vi "Process_NEECA_Data.vi"(4 "Vesta in":refnum<queue>, 7 "Upper Temperature Sensor":T1, 8 "error in (no error)":errorcluster, 9 "VestaTemperature Fixed":T2={"Water Heater Temp (°F)"=125, "Differential  (°F)"=25.0} {"Water Heater Temp (°F)" min=32 max=203}, 10 "Differential_Top":dbl=10.0 format="%#_13g", 11 "Data Cluster":T3={"Vesta Data Output"={"Temp_W_Raw_U"=0, "Temp_W_Raw_L"=0, "Temperature Water (F)"=0.0, "Temperature Water Compensated (F)"=0.0, "Temperature Ambient (F)"=0.0, "Setpoint Location (F)"=0.0, "Heat Request"="", "Fault Ram"="", "PWM DCDC Value"=0, "Pilot Voltage (mV)"=0.0, "Setpoint Actual (F)"=0.0, "Differential Actual (F)"=0.0, "Setpoint User (F)"=0.0, "Differential User (F)"=0.0, "Termperature FIltered -TCO (F)"=0.0, "Temp_C_Raw_1 - Sensor Voltage"="", "Temp_C_Raw_2 - Sensor Voltage"="", "Chamber Sensor Temperature (F)"=0.0, "LDO Base Temperature (F)"=0.0, "LDO Timer (sec)"=0, "Disabled (0)"=FALSE, "Warming (1)"=FALSE, "Heating (2)"=FALSE, "Cooling Data Write (3)"=FALSE, "Cooling (4)"=FALSE, "Data Read (5)"=FALSE, "N/A"=FALSE, "Temperature Trip (7)"=FALSE, "Burner"=FALSE}, "VestaTemperature"={"Water Heater Temp (°F)"=135, "Differential  (°F)"=10.0}, "Timer Application Data"={"Duty Cycle"={"Burner ON Time (Seconds)"=60.0, "Burner OFF Time (Seconds)"=60.0, "Main Burner Flag"=FALSE, "Burner Power Mode"=0, "Off Time Complete Flag"=0, "Heating_Cycle_Released_Flag"=0, "Damper Status"=0, "Damper Burner Seen Flag"=0}}, "Data Array"=[], "MW Output"={"TC1-Channel 021"=0.0, "TC2-Channel 022"=0.0, "TC3-Channel 023"=0.0, "TC4-Channel 024"=0.0, "TC5-Channel 025"=0.0, "TC6-Channel 026"=0.0, "TC7-Channel 017"=0.0, "TC8-Channel 028"=0.0, "TC9-Channel 029"=0.0, "TC10-Channel 030"=0.0, "TC Tree Average"=0.0, "TC DWN- Channel 027"=0.0, "RTDin-Channel 031"=0.0, "RTDout-Channel 032"=0.0, "RTDamb-Channel 033"=0.0, "PSI1-Channel 011"=0.0, "PSI2-Channel 012"=0.0, "PSI3-Channel 013"=0.0, "PSI4-Channel 014"=0.0, "UE State-Channel 015"=0.0, "LE State-Channel 016"=0.0, "Module 4 Relay Status Output"={"INTELLIFAUCET TEMP(T)/FLOW(F) (CH 041)"=FALSE, "INTELLIFAUCET READY (CH 042)"=FALSE, "INTELLIFAUCET START (CH 043)"=FALSE, "INTELLIFAUCET STOP (CH 044)"=FALSE, "MAIN POWER RELAY (CH 047)"=FALSE, "NOT USED (CH 045)"=FALSE, "NOT USED (CH 046)"=FALSE, "PURGE VALVE RELAY (CH 048)"=FALSE, "OUTLET VALVE RELAY (CH 049)"=FALSE, "INLET VALVE RELAY (CH 050)"=FALSE, "Intellifaucet (% Open)"=0.0, "Proportioning Valve (%Open)"=0.0, "Intellifaucet Temp Setpoint (F)"=0.0}}} {"VestaTemperature"."Water Heater Temp (°F)" min=32 max=203}) -> (0 "error out":errorcluster, 2 "Open_Damper":i32, 3 "Data Cluster Output":T3={"Vesta Data Output"={"Temp_W_Raw_U"=0, "Temp_W_Raw_L"=0, "Temperature Water (F)"=0.0, "Temperature Water Compensated (F)"=0.0, "Temperature Ambient (F)"=0.0, "Setpoint Location (F)"=0.0, "Heat Request"="", "Fault Ram"="", "PWM DCDC Value"=0, "Pilot Voltage (mV)"=0.0, "Setpoint Actual (F)"=0.0, "Differential Actual (F)"=0.0, "Setpoint User (F)"=0.0, "Differential User (F)"=0.0, "Termperature FIltered -TCO (F)"=0.0, "Temp_C_Raw_1 - Sensor Voltage"="", "Temp_C_Raw_2 - Sensor Voltage"="", "Chamber Sensor Temperature (F)"=0.0, "LDO Base Temperature (F)"=0.0, "LDO Timer (sec)"=0, "Disabled (0)"=FALSE, "Warming (1)"=FALSE, "Heating (2)"=FALSE, "Cooling Data Write (3)"=FALSE, "Cooling (4)"=FALSE, "Data Read (5)"=FALSE, "N/A"=FALSE, "Temperature Trip (7)"=FALSE, "Burner"=FALSE}, "VestaTemperature"={"Water Heater Temp (°F)"=135, "Differential  (°F)"=10.0}, "Timer Application Data"={"Duty Cycle"={"Burner ON Time (Seconds)"=60.0, "Burner OFF Time (Seconds)"=60.0, "Main Burner Flag"=FALSE, "Burner Power Mode"=0, "Off Time Complete Flag"=0, "Heating_Cycle_Released_Flag"=0, "Damper Status"=0, "Damper Burner Seen Flag"=0}}, "Data Array"=[], "MW Output"={"TC1-Channel 021"=0.0, "TC2-Channel 022"=0.0, "TC3-Channel 023"=0.0, "TC4-Channel 024"=0.0, "TC5-Channel 025"=0.0, "TC6-Channel 026"=0.0, "TC7-Channel 017"=0.0, "TC8-Channel 028"=0.0, "TC9-Channel 029"=0.0, "TC10-Channel 030"=0.0, "TC Tree Average"=0.0, "TC DWN- Channel 027"=0.0, "RTDin-Channel 031"=0.0, "RTDout-Channel 032"=0.0, "RTDamb-Channel 033"=0.0, "PSI1-Channel 011"=0.0, "PSI2-Channel 012"=0.0, "PSI3-Channel 013"=0.0, "PSI4-Channel 014"=0.0, "UE State-Channel 015"=0.0, "LE State-Channel 016"=0.0, "Module 4 Relay Status Output"={"INTELLIFAUCET TEMP(T)/FLOW(F) (CH 041)"=FALSE, "INTELLIFAUCET READY (CH 042)"=FALSE, "INTELLIFAUCET START (CH 043)"=FALSE, "INTELLIFAUCET STOP (CH 044)"=FALSE, "MAIN POWER RELAY (CH 047)"=FALSE, "NOT USED (CH 045)"=FALSE, "NOT USED (CH 046)"=FALSE, "PURGE VALVE RELAY (CH 048)"=FALSE, "OUTLET VALVE RELAY (CH 049)"=FALSE, "INLET VALVE RELAY (CH 050)"=FALSE, "Intellifaucet (% Open)"=0.0, "Proportioning Valve (%Open)"=0.0, "Intellifaucet Temp Setpoint (F)"=0.0}}} {"VestaTemperature"."Water Heater Temp (°F)" min=32 max=203})   [LabVIEW 2023]
uses:
  Message Queue/Message Cluster.ctl
  controls/UI Data.ctl
  Drivers/Resideo Gas Valve/Type Definitions/Vesta Info.ctl
  Drivers/Resideo Gas Valve/Type Definitions/Temperature Control.ctl
  controls/Timer Application Cluster.ctl
  controls/Burner Duty Cycle.ctl
  Hybrid Water Heater/Type Definitions/HEWH MW100 Data Cluster.ctl
  Hybrid Water Heater/Custom Instrument Control/MW100/Type Definitions/HEWH Module 4 Relay Status.ctl
  controls/Upper Temperature Sensor.ctl
  <vilib>/Utility/error.llb/whitespace.ctl
  <vilib>/Utility/error.llb/Trim Whitespace One-Sided.vi
  Message Queue/Message Queue.lvlib
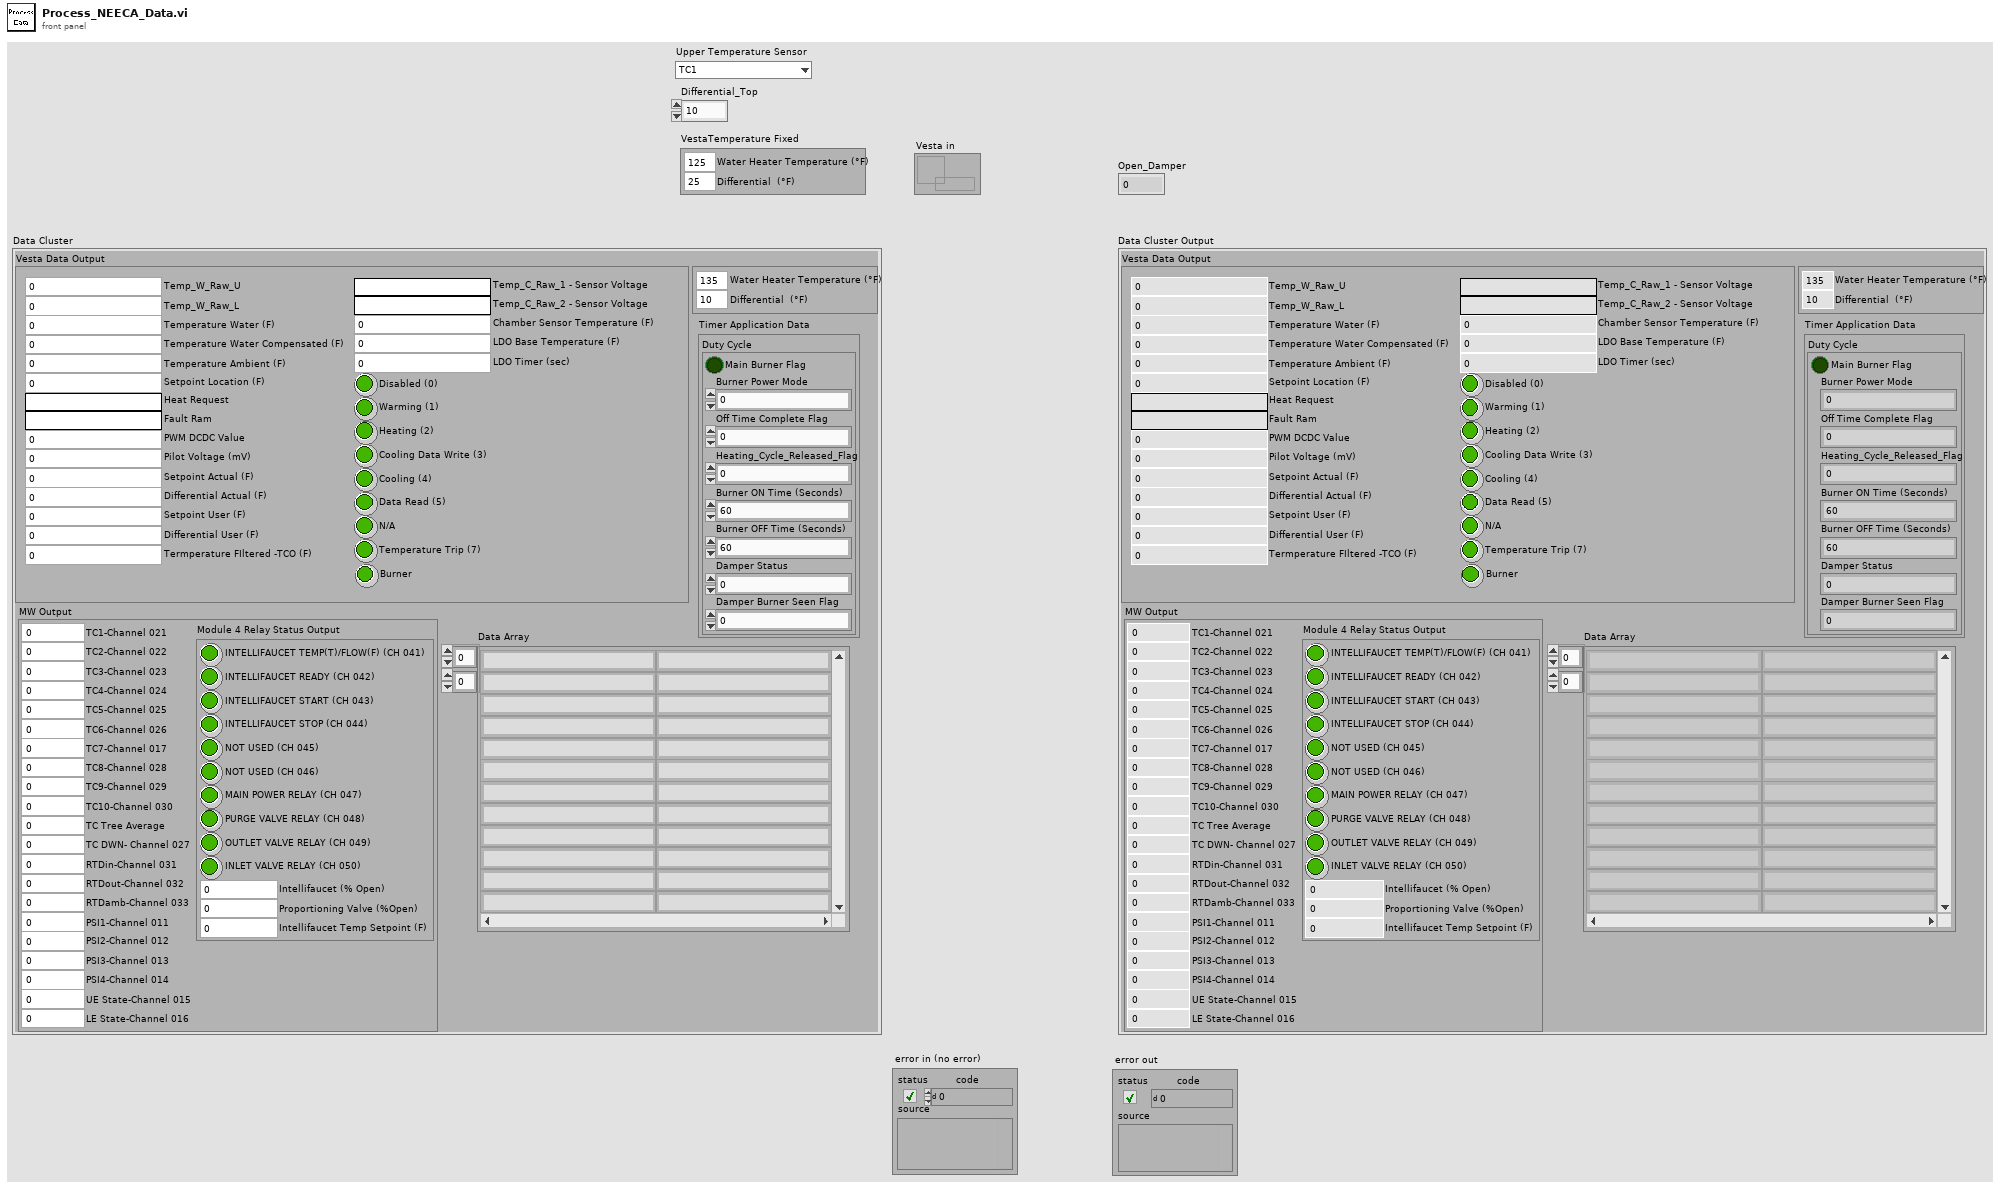
[diagram p1: front panel]
types:
  T1 = typedef "Upper Temperature Sensor.ctl" = enum16{"TC1", "TC2", "TC3", "TC4", "TC5", "TC6"}
  T2 = typedef "Temperature Control.ctl" = cluster{"Water Heater Temp (°F)":u16, "Differential  (°F)":dbl}
  T3 = typedef "UI Data.ctl" = cluster{"Vesta Data Output":T4, "VestaTemperature":T2, "Timer Application Data":T5, "Data Array":string[][], "MW Output":T7}
  T4 = typedef "Vesta Info.ctl" = cluster{"Temp_W_Raw_U":u16, "Temp_W_Raw_L":u16, "Temperature Water (F)":dbl, "Temperature Water Compensated (F)":dbl, "Temperature Ambient (F)":dbl, "Setpoint Location (F)":dbl, "Heat Request":string, "Fault Ram":string, "PWM DCDC Value":u16, "Pilot Voltage (mV)":dbl, "Setpoint Actual (F)":dbl, "Differential Actual (F)":dbl, "Setpoint User (F)":dbl, "Differential User (F)":dbl, "Termperature FIltered -TCO (F)":dbl, "Temp_C_Raw_1 - Sensor Voltage":string, "Temp_C_Raw_2 - Sensor Voltage":string, "Chamber Sensor Temperature (F)":dbl, "LDO Base Temperature (F)":dbl, "LDO Timer (sec)":i16, "Disabled (0)":bool, "Warming (1)":bool, "Heating (2)":bool, "Cooling Data Write (3)":bool, "Cooling (4)":bool, "Data Read (5)":bool, "N/A":bool, "Temperature Trip (7)":bool, "Burner":bool}
  T5 = typedef "Timer Application Cluster.ctl" = cluster{"Duty Cycle":T6}
  T6 = typedef "Burner Duty Cycle.ctl" = cluster{"Burner ON Time (Seconds)":dbl, "Burner OFF Time (Seconds)":dbl, "Main Burner Flag":bool, "Burner Power Mode":u8, "Off Time Complete Flag":u8, "Heating_Cycle_Released_Flag":u8, "Damper Status":u8, "Damper Burner Seen Flag":u8}
  T7 = typedef "HEWH MW100 Data Cluster.ctl" = cluster{"TC1-Channel 021":dbl, "TC2-Channel 022":dbl, "TC3-Channel 023":dbl, "TC4-Channel 024":dbl, "TC5-Channel 025":dbl, "TC6-Channel 026":dbl, "TC7-Channel 017":dbl, "TC8-Channel 028":dbl, "TC9-Channel 029":dbl, "TC10-Channel 030":dbl, "TC Tree Average":dbl, "TC DWN- Channel 027":dbl, "RTDin-Channel 031":dbl, "RTDout-Channel 032":dbl, "RTDamb-Channel 033":dbl, "PSI1-Channel 011":dbl, "PSI2-Channel 012":dbl, "PSI3-Channel 013":dbl, "PSI4-Channel 014":dbl, "UE State-Channel 015":dbl, "LE State-Channel 016":dbl, "Module 4 Relay Status Output":T8}
  T8 = typedef "HEWH Module 4 Relay Status.ctl" = cluster{"INTELLIFAUCET TEMP(T)/FLOW(F) (CH 041)":bool, "INTELLIFAUCET READY (CH 042)":bool, "INTELLIFAUCET START (CH 043)":bool, "INTELLIFAUCET STOP (CH 044)":bool, "MAIN POWER RELAY (CH 047)":bool, "NOT USED (CH 045)":bool, "NOT USED (CH 046)":bool, "PURGE VALVE RELAY (CH 048)":bool, "OUTLET VALVE RELAY (CH 049)":bool, "INLET VALVE RELAY (CH 050)":bool, "Intellifaucet (% Open)":dbl, "Proportioning Valve (%Open)":dbl, "Intellifaucet Temp Setpoint (F)":dbl}
  T9 = typedef "whitespace.ctl" = u16
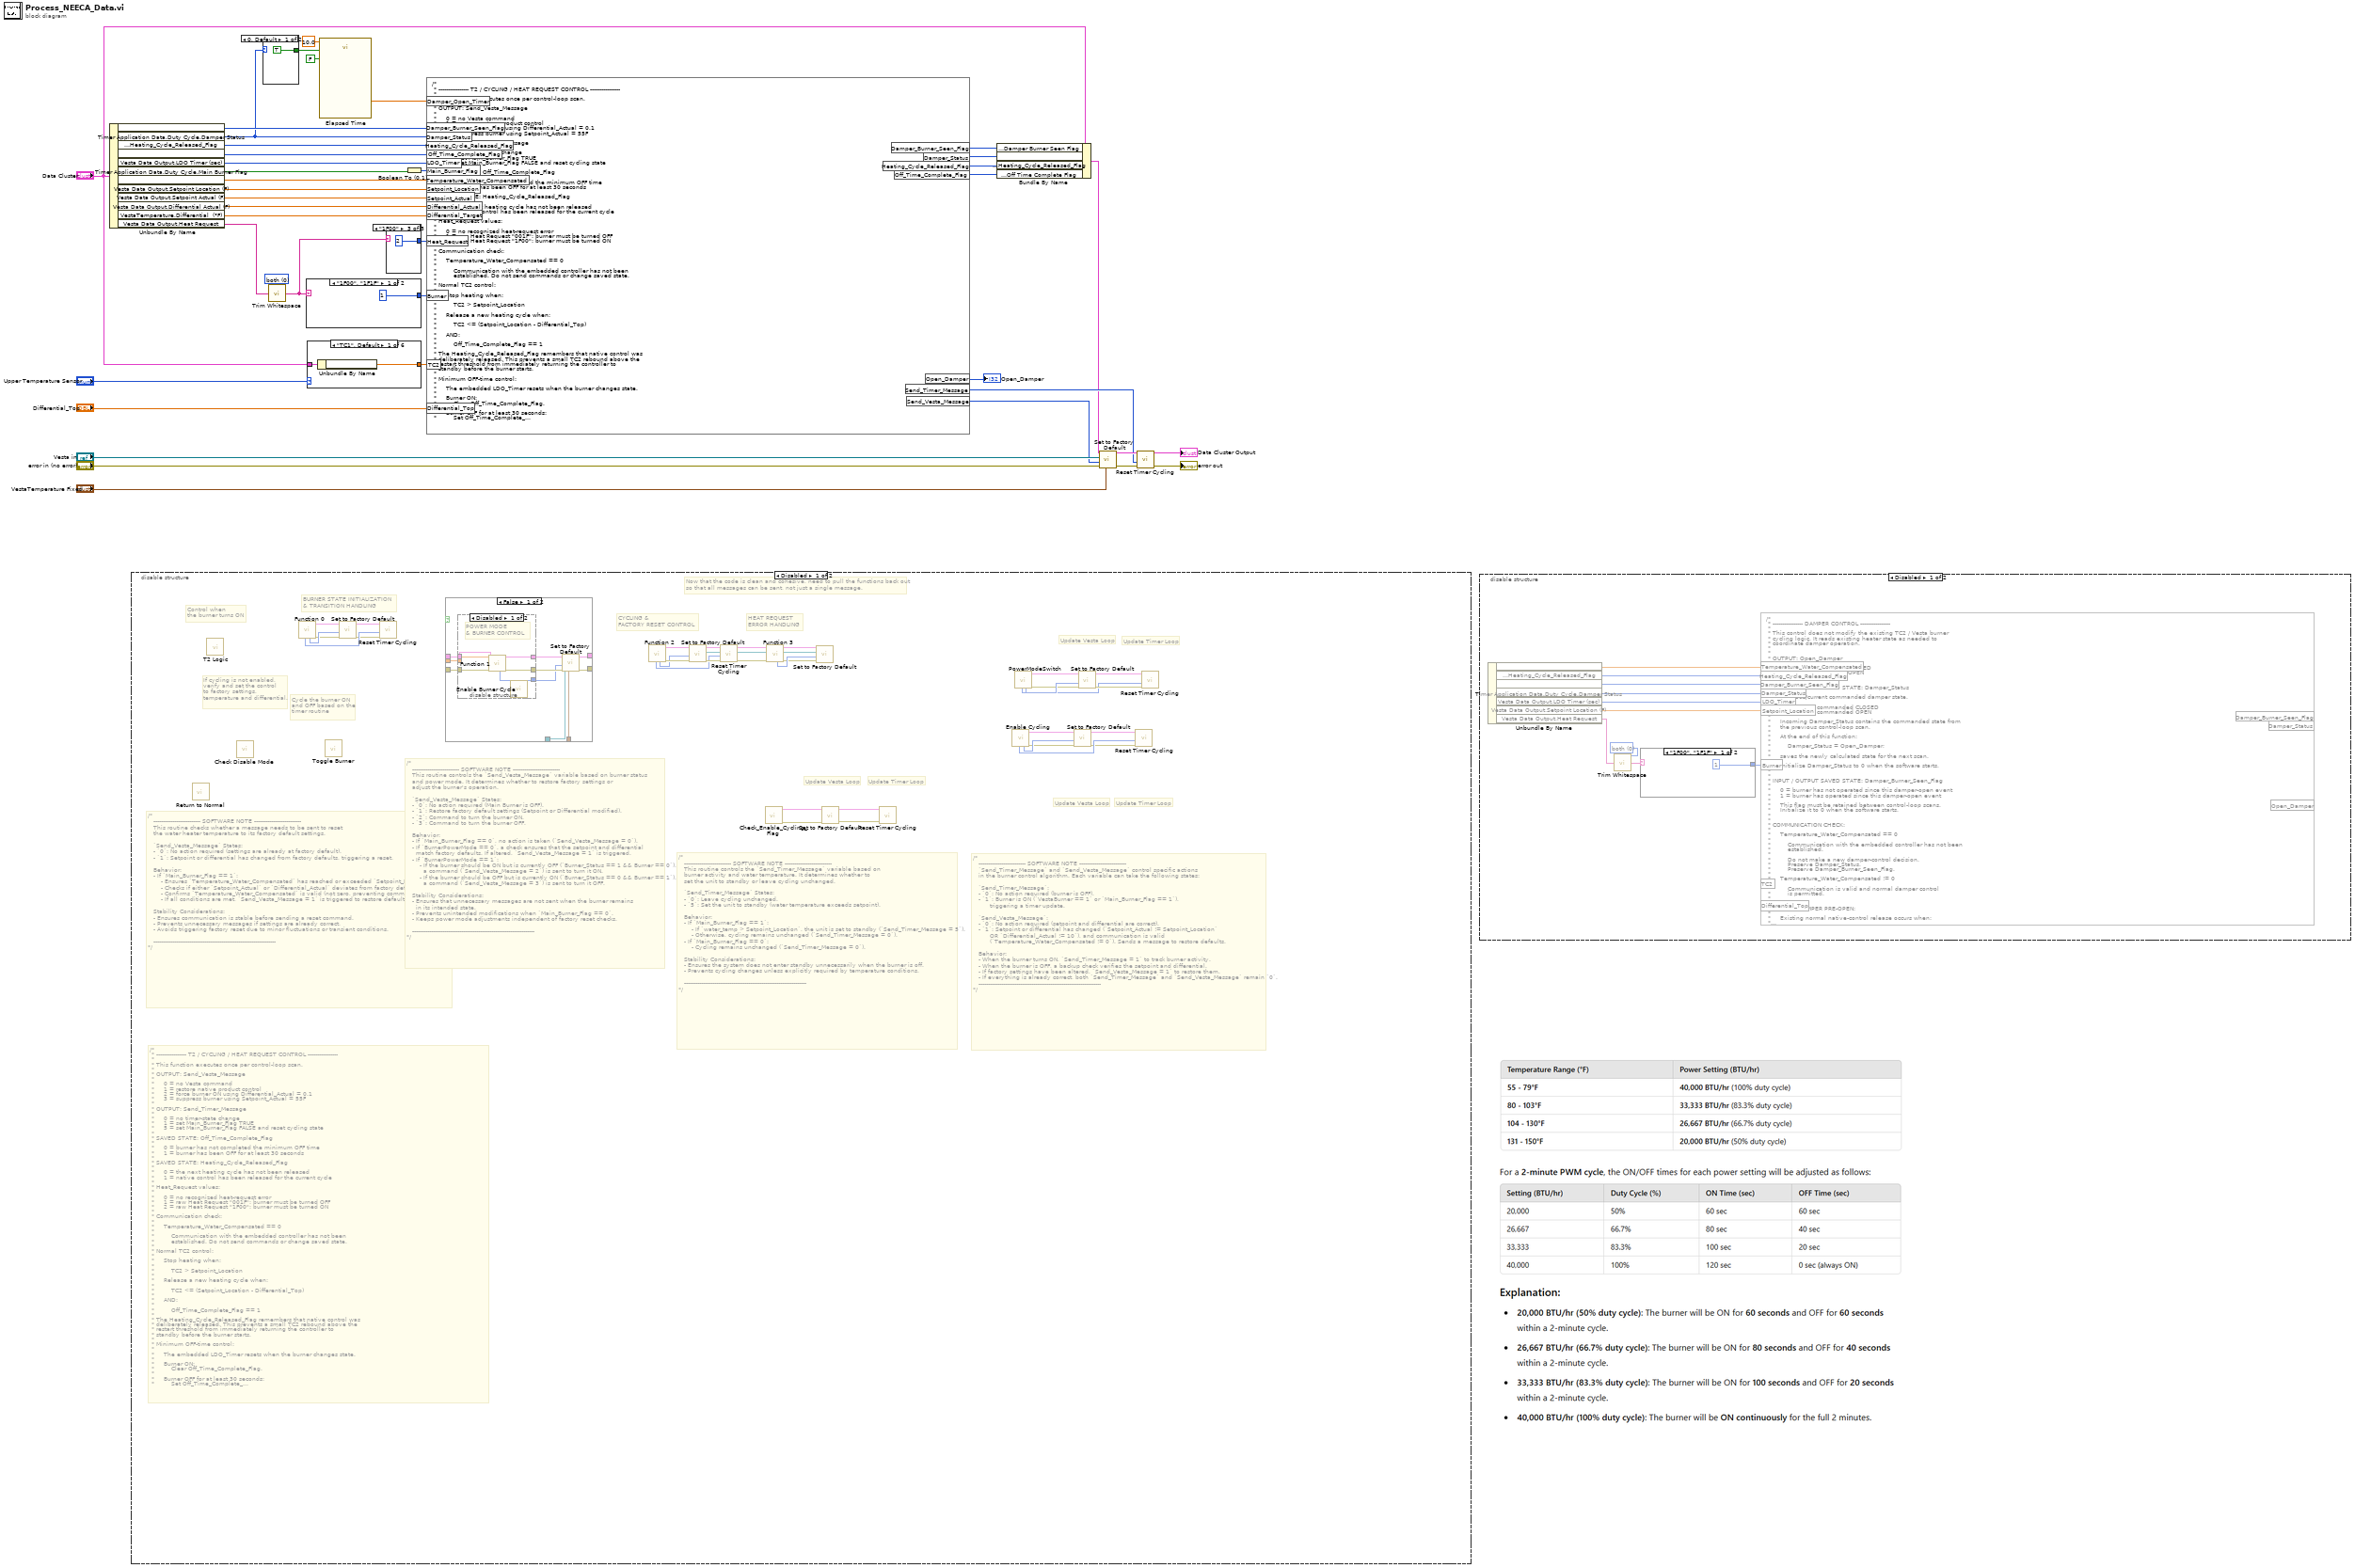
[diagram p0: block diagram]
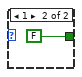
[diagram p2: hidden frame]
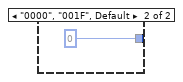
[diagram p3: hidden frame]
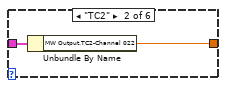
[diagram p5: hidden frame]
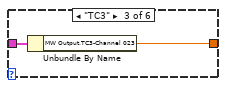
[diagram p6: hidden frame]
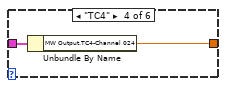
[diagram p7: hidden frame]
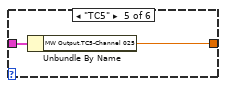
[diagram p8: hidden frame]
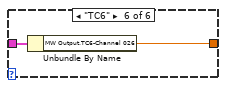
[diagram p9: hidden frame]
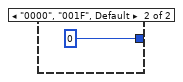
[diagram p10: hidden frame]
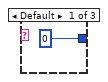
[diagram p11: hidden frame]
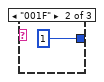
[diagram p12: hidden frame]
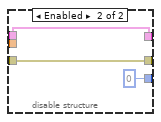
[diagram p13: hidden frame]
diagram:
  w27 = T9 0 items=["both", "start of string", "end of string"] ("location (both)")
  n1 = Unbundle By Name("Data Cluster") -> ("Timer Application Data.Duty Cycle.Damper Burner Seen Flag"=w9:u8, "Timer Application Data.Duty Cycle.Damper Status"=w3:u8, "Timer Application Data.Duty Cycle.Heating_Cycle_Released_Flag"=w14:u8, "Timer Application Data.Duty Cycle.Off Time Complete Flag"=w18:u8, "Vesta Data Output.LDO Timer (sec)"=w19:i16, "Timer Application Data.Duty Cycle.Main Burner Flag"=w24:bool, "Vesta Data Output.Temperature Water Compensated (F)"=w36:dbl, "Vesta Data Output.Setpoint Location (F)"=w31:dbl, "Vesta Data Output.Setpoint Actual (F)"=w30:dbl, "Vesta Data Output.Differential Actual (F)"=w29:dbl, "VestaTemperature.Differential  (°F)"=w28:dbl, "Vesta Data Output.Heat Request"=w26:string)
  n2 = disable-structure shown="Disabled" {
    frame Disabled {
      # "/*\n * ---------------- T2 / CYCLING / HEAT REQUEST CONTROL ----------------\n *\n * This function executes once per control-loop scan.\n *\n * OUTPUT: Send_Vesta_Message\n *\n *     0 = no Vesta command\n *     1 = restore native product control\n *     2 = force burner ON using Differential_Actual = 0.1\n *     3 = suppress burner using Setpoint_Actual = 55F\n *\n * OUTPUT: Send_Timer_Message\n *\n *     0 = no timer-state change\n *     1 = set Main_Burner_Flag TRUE\n *     5 = set Main_Burner_Flag FALSE and reset cycling state\n *\n * SAVED STATE: Off_Time_Complete_Flag\n *\n *     0 = burner has not completed the minimum OFF time\n *     1 = burner has been OFF for at least 30 seconds\n *\n * SAVED STATE: Heating_Cycle_Released_Flag\n *\n *     0 = the next heating cycle has not been released\n *     1 = native control has been released for the current cycle\n *\n * Heat_Request values:\n *\n *     0 = no recognized heat-request error\n *     1 = raw Heat Request \"001F\": burner must be turned OFF\n *     2 = raw Heat Request \"1F00\": burner must be turned ON\n *\n * Communication check:\n *\n *     Temperature_Water_Compensated == 0\n *\n *         Communication with the embedded controller has not been\n *         established. Do not send commands or change saved state.\n *\n * Normal TC2 control:\n *\n *     Stop heating when:\n *\n *         TC2 > Setpoint_Location\n *\n *     Release a new heating cycle when:\n *\n *         TC2 <= (Setpoint_Location - Differential_Top)\n *\n *     AND:\n *\n *         Off_Time_Complete_Flag == 1\n *\n * The Heating_Cycle_Released_Flag remembers that native control was\n * deliberately released. This prevents a small TC2 rebound above the\n * restart threshold from immediately returning the controller to\n * standby before the burner starts.\n *\n * Minimum OFF-time control:\n *\n *     The embedded LDO_Timer resets when the burner changes state.\n *\n *     Burner ON:\n *         Clear Off_Time_Complete_Flag.\n *\n *     Burner OFF for at least 30 seconds:\n *         Set Off_Time_Complete_Flag.\n *\n *     Once set, the flag stays set throughout the same OFF period.\n *     This prevents LDO_Timer rollover from restarting the lockout.\n *\n * Forced-ON error recovery:\n *\n *     Heat_Request == 2 applies Differential_Actual = 0.1.\n *\n *     After Heat_Request returns to zero, remove the 0.1 differential\n *     immediately. Do not wait for the TC2 restart threshold or the\n *     30-second OFF-time requirement.\n *\n * Control priority:\n *\n *     0. Embedded communication check\n *     1. Active Heat Request error handling\n *     2. Residual forced-ON error recovery\n *     3. Pilot position\n *     4. Normal TC2 cycle-release control\n */\n\n\n/* ---------------- Output defaults ---------------- */\n\nint32 Send_Vesta_Message = 0;\nint32 Send_Timer_Message = 0;\nint32 Open_Damper = 0;\n\n\n/* ---------------- Controller-state variables ---------------- */\n\nint32 native_controls_active = 0;\nint32 standby_is_active = 0;\nint32 forced_on_is_active = 0;\n\n\n/* ---------------- Communication and TC2 variables ---------------- */\n\nint32 lower_temperature_valid = 0;\nint32 upper_is_high = 0;\nint32 upper_restart_allowed = 0;\n\n\n/* ---------------- Previous saved-state values ---------------- */\n\nint32 Off_Time_Complete_Flag_Previous = 0;\nint32 Heating_Cycle_Released_Flag_Previous = 0;\n\n\n/* ---------------- Constants ---------------- */\n\nfloat Pilot_Position = 0.1;\nfloat Forced_On_Differential = 0.1;\n\nint32 LDO_Timeout_OFF = 30;\n\n\n/* ---------------- Decoded Heat Request values ---------------- */\n\nint32 Heat_Request_None = 0;\nint32 Heat_Request_Turn_Off = 1;  /* Raw value \"001F\" */\nint32 Heat_Request_Turn_On = 2;   /* Raw value \"1F00\" */\n\n\n/* ================================================================\n * SAVE INCOMING STATE VALUES\n * ================================================================ */\n\n/*\n * Both saved-state variables are Formula Node inputs and outputs.\n *\n * Preserve the incoming values by default. The control logic below\n * changes them only when a defined state transition occurs.\n */\n\nOff_Time_Complete_Flag_Previous =\n    Off_Time_Complete_Flag;\n\nHeating_Cycle_Released_Flag_Previous =\n    Heating_Cycle_Released_Flag;\n\nOff_Time_Complete_Flag =\n    Off_Time_Complete_Flag_Previous;\n\nHeating_Cycle_Released_Flag =\n    Heating_Cycle_Released_Flag_Previous;\n\n\n/* ================================================================\n * DETERMINE CURRENT EMBEDDED CONTROLLER STATE\n * ================================================================ */\n\n/*\n * Native control:\n *\n *     Setpoint_Actual = physical knob setting\n *     Differential_Actual = normal embedded differential\n */\n\nnative_controls_active =\n    ((Setpoint_Actual == Setpoint_Location) &&\n     (Differential_Actual == Differential_Target)) ? 1 : 0;\n\n\n/*\n * Standby:\n *\n *     Setpoint_Actual = 55F\n *     Differential_Actual = normal embedded differential\n */\n\nstandby_is_active =\n    ((Setpoint_Actual == 55.0) &&\n     (Differential_Actual == Differential_Target)) ? 1 : 0;\n\n\n/*\n * Forced ON:\n *\n *     Setpoint_Actual = physical knob setting\n *     Differential_Actual = 0.1\n */\n\nforced_on_is_active =\n    ((Setpoint_Actual == Setpoint_Location) &&\n     (Differential_Actual == Forced_On_Differential)) ? 1 : 0;\n\n\n/* ================================================================\n * DETERMINE COMMUNICATION STATUS\n * ================================================================ */\n\n/*\n * Temperature_Water_Compensated is used only as the communication\n * check in this function.\n *\n * A value of zero indicates that a valid reading has not been\n * received from the embedded controller.\n */\n\nlower_temperature_valid =\n    (Temperature_Water_Compensated == 0) ? 0 : 1;\n\n\n/* ================================================================\n * DETERMINE TC2 CONDITIONS\n * ================================================================ */\n\n/*\n * Stop heating when TC2 rises above the physical knob setpoint.\n *\n * At exact equality, upper_is_high remains zero.\n */\n\nupper_is_high =\n    (TC2 > Setpoint_Location) ? 1 : 0;\n\n\n/*\n * Permit release of a new heating cycle after TC2 cools to or below:\n *\n *     Setpoint_Location - Differential_Top\n *\n * Example:\n *\n *     Setpoint_Location = 125F\n *     Differential_Top = 5F\n *\n *     Stop threshold:    TC2 > 125F\n *     Restart threshold: TC2 <= 120F\n */\n\nupper_restart_allowed =\n    (TC2 <=\n        (Setpoint_Location - Differential_Top)) ? 1 : 0;\n\n\n/* ================================================================\n * PRIORITY 0: EMBEDDED COMMUNICATION CHECK\n * ================================================================ */\n\nif (lower_temperature_valid == 0)\n{\n    /*\n     * Communication has not been established.\n     *\n     * Do not send Vesta commands.\n     * Do not send timer commands.\n     * Do not change either saved-state flag.\n     */\n\n    Send_Vesta_Message = 0;\n    Send_Timer_Message = 0;\n\n    Off_Time_Complete_Flag =\n        Off_Time_Complete_Flag_Previous;\n\n    Heating_Cycle_Released_Flag =\n        Heating_Cycle_Released_Flag_Previous;\n}\n\n\n/* ================================================================\n * COMMUNICATION IS VALID\n * ================================================================ */\n\nelse\n{\n    /* ------------------------------------------------------------\n     * UPDATE MINIMUM OFF-TIME STATE\n     * ------------------------------------------------------------ */\n\n    /*\n     * Burner ON:\n     *\n     * The burner is no longer in an OFF period. Clear the completed\n     * OFF-time flag.\n     */\n\n    if (Burner == 1)\n    {\n        Off_Time_Complete_Flag = 0;\n    }\n\n\n    /*\n     * Burner OFF:\n     *\n     * Set the completed flag after LDO_Timer reaches 30 seconds.\n     *\n     * Once set, preserve the flag throughout the same OFF period.\n     * LDO_Timer may later roll over, but the saved flag stays set.\n     */\n\n    else if (Burner == 0)\n    {\n        if (Off_Time_Complete_Flag_Previous == 0)\n        {\n            if (LDO_Timer >= LDO_Timeout_OFF)\n            {\n                Off_Time_Complete_Flag = 1;\n            }\n        }\n    }\n\n\n    /*\n     * Unexpected burner value:\n     *\n     * Preserve the previous OFF-time state.\n     */\n\n    else\n    {\n        Off_Time_Complete_Flag =\n            Off_Time_Complete_Flag_Previous;\n    }\n\n\n    /* ============================================================\n     * PRIORITY 1A: ACTIVE TURN-OFF ERROR\n     * ============================================================ */\n\n    /*\n     * Heat_Request == 1 corresponds to raw value \"001F\".\n     *\n     * The error condition requires the burner to be turned OFF.\n     */\n\n    if (Heat_Request == Heat_Request_Turn_Off)\n    {\n        /*\n         * Immediately command 55F standby.\n         *\n         * Vesta message 3 also restores:\n         *\n         *     Differential_Actual = Differential_Target\n         */\n\n        if (standby_is_active == 0)\n        {\n            Send_Vesta_Message = 3;\n        }\n\n        /*\n         * Withdraw normal-cycle permission.\n         *\n         * After the error clears, the next normal cycle must satisfy\n         * the TC2 restart and minimum OFF-time requirements.\n         */\n\n        Heating_Cycle_Released_Flag = 0;\n\n        /*\n         * Do not clear Main_Burner_Flag until Burner == 0 confirms\n         * that the burner has physically shut down.\n         */\n    }\n\n\n    /* ============================================================\n     * PRIORITY 1B: ACTIVE FORCED-ON ERROR\n     * ============================================================ */\n\n    /*\n     * Heat_Request == 2 corresponds to raw value \"1F00\".\n     *\n     * The error condition requires the burner to be turned ON.\n     */\n\n    else if (Heat_Request == Heat_Request_Turn_On)\n    {\n        /*\n         * Immediately apply the 0.1 embedded lower differential.\n         *\n         * Active error handling is not delayed by TC2 restart\n         * permission or the 30-second minimum OFF time.\n         */\n\n        if (forced_on_is_active == 0)\n        {\n            Send_Vesta_Message = 2;\n        }\n\n        /*\n         * Preserve Heating_Cycle_Released_Flag while the active error\n         * is present.\n         *\n         * The residual forced-ON recovery below determines the proper\n         * normal state after Heat_Request returns to zero.\n         */\n    }\n\n\n    /* ============================================================\n     * PRIORITY 2: NO ACTIVE HEAT REQUEST ERROR\n     * ============================================================ */\n\n    else if (Heat_Request == Heat_Request_None)\n    {\n        /* --------------------------------------------------------\n         * RESIDUAL FORCED-ON ERROR RECOVERY\n         * -------------------------------------------------------- */\n\n        /*\n         * Heat_Request has cleared, but the controller still reports:\n         *\n         *     Setpoint_Actual = Setpoint_Location\n         *     Differential_Actual = 0.1\n         *\n         * Remove the 0.1 differential immediately.\n         *\n         * Do not wait for:\n         *\n         *     upper_restart_allowed\n         *     Off_Time_Complete_Flag\n         */\n\n        if (forced_on_is_active == 1)\n        {\n            /*\n             * TC2 is above the customer setpoint.\n             *\n             * Enter standby immediately and withdraw heating-cycle\n             * permission.\n             */\n\n            if (upper_is_high == 1)\n            {\n                Send_Vesta_Message = 3;\n                Heating_Cycle_Released_Flag = 0;\n            }\n\n\n            /*\n             * TC2 is not above the customer setpoint.\n             *\n             * Immediately restore:\n             *\n             *     Setpoint_Actual = Setpoint_Location\n             *     Differential_Actual = Differential_Target\n             *\n             * Consider the current cycle released. The embedded lower\n             * thermistor then decides whether the burner continues,\n             * shuts off, or starts later.\n             */\n\n            else\n            {\n                Send_Vesta_Message = 1;\n                Heating_Cycle_Released_Flag = 1;\n            }\n\n\n            /*\n             * Synchronize Main_Burner_Flag with the physical burner.\n             */\n\n            if (Burner == 1)\n            {\n                if (Main_Burner_Flag == 0)\n                {\n                    Send_Timer_Message = 1;\n                }\n            }\n\n            else if (Burner == 0)\n            {\n                if (Main_Burner_Flag == 1)\n                {\n                    Send_Timer_Message = 5;\n                }\n            }\n        }\n\n\n        /* --------------------------------------------------------\n         * USER-SELECTED PILOT POSITION\n         * -------------------------------------------------------- */\n\n        else if (Setpoint_Location == Pilot_Position)\n        {\n            /*\n             * Pilot was selected using the physical product control.\n             *\n             * Do not send Vesta or timer commands.\n             * Withdraw normal heating-cycle permission so that the\n             * control initializes again after leaving Pilot.\n             */\n\n            Send_Vesta_Message = 0;\n            Send_Timer_Message = 0;\n\n            Heating_Cycle_Released_Flag = 0;\n        }\n\n\n        /* --------------------------------------------------------\n         * BURNER ON\n         * -------------------------------------------------------- */\n\n        else if (Burner == 1)\n        {\n            /*\n             * TC2 is above the physical knob setpoint.\n             *\n             * Stop heating immediately regardless of release state.\n             */\n\n            if (upper_is_high == 1)\n            {\n                if (standby_is_active == 0)\n                {\n                    Send_Vesta_Message = 3;\n                }\n\n                /*\n                 * Withdraw permission for the next heating cycle.\n                 */\n\n                Heating_Cycle_Released_Flag = 0;\n\n                /*\n                 * Do not clear Main_Burner_Flag yet.\n                 *\n                 * Wait for Burner == 0 to confirm physical shutdown.\n                 */\n            }\n\n\n            /*\n             * A normal cycle was previously released.\n             *\n             * Continue heating while TC2 remains at or below the\n             * upper stopping threshold.\n             */\n\n            else if (Heating_Cycle_Released_Flag_Previous == 1)\n            {\n                Heating_Cycle_Released_Flag = 1;\n\n                if (Main_Burner_Flag == 0)\n                {\n                    Send_Timer_Message = 1;\n                }\n            }\n\n\n            /*\n             * Burner is already ON, but no released cycle has yet\n             * been recorded.\n             *\n             * This can happen during:\n             *\n             *     Cold-tank startup\n             *     Software restart\n             *     State recovery\n             *\n             * Adopt the active cycle only when TC2 is already at or\n             * below the normal restart threshold.\n             */\n\n            else\n            {\n                if (upper_restart_allowed == 1)\n                {\n                    /*\n                     * Adopt the valid cold-start heating cycle.\n                     */\n\n                    Heating_Cycle_Released_Flag = 1;\n\n                    /*\n                     * If the controller is not already in native mode,\n                     * restore native settings.\n                     */\n\n                    if (native_controls_active == 0)\n                    {\n                        Send_Vesta_Message = 1;\n                    }\n\n                    if (Main_Burner_Flag == 0)\n                    {\n                        Send_Timer_Message = 1;\n                    }\n                }\n\n\n                /*\n                 * The burner is ON, but TC2 is still above the restart\n                 * threshold.\n                 *\n                 * Do not adopt this cycle. Command standby and keep the\n                 * cycle locked out.\n                 */\n\n                else\n                {\n                    if (standby_is_active == 0)\n                    {\n                        Send_Vesta_Message = 3;\n                    }\n\n                    Heating_Cycle_Released_Flag = 0;\n                }\n            }\n        }\n\n\n        /* --------------------------------------------------------\n         * BURNER OFF\n         * -------------------------------------------------------- */\n\n        else if (Burner == 0)\n        {\n            /*\n             * Clear Main_Burner_Flag only after physical burner\n             * shutdown is confirmed.\n             */\n\n            if (Main_Burner_Flag == 1)\n            {\n                Send_Timer_Message = 5;\n            }\n\n\n            /*\n             * A cycle was previously released.\n             */\n\n            if (Heating_Cycle_Released_Flag_Previous == 1)\n            {\n                /*\n                 * TC2 has exceeded the customer setpoint while the\n                 * burner is OFF.\n                 *\n                 * Enter standby and close the released cycle.\n                 */\n\n                if (upper_is_high == 1)\n                {\n                    if (standby_is_active == 0)\n                    {\n                        Send_Vesta_Message = 3;\n                    }\n\n                    Heating_Cycle_Released_Flag = 0;\n                }\n\n\n                /*\n                 * Main_Burner_Flag is still one while Burner is zero.\n                 *\n                 * The embedded controller has just ended an active\n                 * burner cycle. Enter standby and require the next\n                 * cycle to satisfy TC2 and minimum OFF-time criteria.\n                 */\n\n                else if (Main_Burner_Flag == 1)\n                {\n                    if (standby_is_active == 0)\n                    {\n                        Send_Vesta_Message = 3;\n                    }\n\n                    Heating_Cycle_Released_Flag = 0;\n                }\n\n\n                /*\n                 * The cycle has been released, but the burner has not\n                 * started yet.\n                 *\n                 * Keep native control released while waiting for the\n                 * embedded lower thermistor to call for heat.\n                 *\n                 * Do not cancel the release merely because TC2 rises\n                 * slightly above the restart threshold.\n                 */\n\n                else\n                {\n                    Heating_Cycle_Released_Flag = 1;\n\n                    /*\n                     * If message 1 has not yet been acknowledged and\n                     * standby still reports active, repeat the same\n                     * release command. Do not issue an opposing\n                     * standby command.\n                     */\n\n                    if (standby_is_active == 1)\n                    {\n                        Send_Vesta_Message = 1;\n                    }\n\n                    else\n                    {\n                        Send_Vesta_Message = 0;\n                    }\n                }\n            }\n\n\n            /*\n             * No heating cycle is currently released.\n             */\n\n            else\n            {\n                /*\n                 * TC2 is above the physical knob setpoint.\n                 *\n                 * Ensure the controller is in standby.\n                 */\n\n                if (upper_is_high == 1)\n                {\n                    if (standby_is_active == 0)\n                    {\n                        Send_Vesta_Message = 3;\n                    }\n\n                    Heating_Cycle_Released_Flag = 0;\n                }\n\n\n                /*\n                 * The controller already reports standby.\n                 *\n                 * Release native control only after:\n                 *\n                 *     1. TC2 reaches the restart threshold.\n                 *     2. Burner has been OFF for at least 30 seconds.\n                 */\n\n                else if (standby_is_active == 1)\n                {\n                    if ((upper_restart_allowed == 1) &&\n                        (Off_Time_Complete_Flag == 1))\n                    {\n                        Send_Vesta_Message = 1;\n                        Heating_Cycle_Released_Flag = 1;\n                    }\n\n                    else\n                    {\n                        Send_Vesta_Message = 0;\n                        Heating_Cycle_Released_Flag = 0;\n                    }\n                }\n\n\n                /*\n                 * The controller reports native mode, but the cycle\n                 * has not yet been released.\n                 *\n                 * This is the startup and state-initialization case.\n                 */\n\n                else if (native_controls_active == 1)\n                {\n                    /*\n                     * Cold start or sufficiently cooled tank:\n                     *\n                     * Native control may remain active only after the\n                     * TC2 and minimum OFF-time criteria are satisfied.\n                     */\n\n                    if ((upper_restart_allowed == 1) &&\n                        (Off_Time_Complete_Flag == 1))\n                    {\n                        Send_Vesta_Message = 0;\n                        Heating_Cycle_Released_Flag = 1;\n                    }\n\n\n                    /*\n                     * Hot startup or minimum OFF time not complete:\n                     *\n                     * Place the controller into standby and lock out\n                     * the next heating cycle.\n                     */\n\n                    else\n                    {\n                        Send_Vesta_Message = 3;\n                        Heating_Cycle_Released_Flag = 0;\n                    }\n                }\n\n\n                /*\n                 * The applied state does not match native or standby.\n                 *\n                 * This may occur while a previous Vesta command is\n                 * still being processed. Do not issue an opposing\n                 * command.\n                 */\n\n                else\n                {\n                    Send_Vesta_Message = 0;\n                    Heating_Cycle_Released_Flag = 0;\n                }\n            }\n        }\n\n\n        /* --------------------------------------------------------\n         * UNEXPECTED BURNER VALUE\n         * -------------------------------------------------------- */\n\n        else\n        {\n            Send_Vesta_Message = 0;\n            Send_Timer_Message = 0;\n\n            Heating_Cycle_Released_Flag =\n                Heating_Cycle_Released_Flag_Previous;\n        }\n    }\n\n\n    /* ============================================================\n     * UNEXPECTED HEAT REQUEST VALUE\n     * ============================================================ */\n\n    else\n    {\n        Send_Vesta_Message = 0;\n        Send_Timer_Message = 0;\n\n        Heating_Cycle_Released_Flag =\n            Heating_Cycle_Released_Flag_Previous;\n    }\n}"
      # "Control when\nthe burner turns ON"
      # "CYCLING &\nFACTORY RESET CONTROL"
      # "HEAT REQUEST\nERROR HANDLING"
      # "BURNER STATE INITIALIZATION\n& TRANSITION HANDLING"
      # "Update Timer Loop"
      # "Update Vesta Loop"
      # "Now that the code is clean and cohesive, need to pull the functions back out\nso that all messages can be sent, not just a single message."
      # "/*  \n   ------------------------- SOFTWARE NOTE -------------------------  \n   `Send_Timer_Message` and `Send_Vesta_Message` control specific actions  \n   in the burner control algorithm. Each variable can take the following states:  \n\n   `Send_Timer_Message`:  \n   - `0`: No action required (burner is OFF).  \n   - `1`: Burner is ON (`VestaBurner == 1` or `Main_Burner_Flag == 1`),  \n         triggering a timer update.  \n\n   `Send_Vesta_Message`:  \n   - `0`: No action required (setpoint and differential are correct).  \n   - `1`: Setpoint or differential has changed (`Setpoint_Actual != Setpoint_Location`  \n         OR `Differential_Actual != 10`), and communication is valid  \n         (`Temperature_Water_Compensated != 0`). Sends a message to restore defaults.  \n\n   Behavior:  \n   - When the burner turns ON, `Send_Timer_Message = 1` to track burner activity.  \n   - When the burner is OFF, a backup check verifies the setpoint and differential.  \n   - If factory settings have been altered, `Send_Vesta_Message = 1` to restore them.  \n   - If everything is already correct, both `Send_Timer_Message` and `Send_Vesta_Message` remain `0`.  \n   -----------------------------------------------------------------  \n*/"
      # "Update Timer Loop"
      # "Update Vesta Loop"
      # "Update Timer Loop"
      # "Update Vesta Loop"
      # "/*  \n   ------------------------- SOFTWARE NOTE -------------------------  \n   This routine controls the `Send_Timer_Message` variable based on  \n   burner activity and water temperature. It determines whether to  \n   set the unit to standby or leave cycling unchanged.\n\n   `Send_Timer_Message` States:  \n   - `0`: Leave cycling unchanged.  \n   - `5`: Set the unit to standby (water temperature exceeds setpoint).  \n\n   Behavior:  \n   - If `Main_Burner_Flag == 1`:  \n       - If `water_temp > Setpoint_Location`, the unit is set to standby (`Send_Timer_Message = 5`).  \n       - Otherwise, cycling remains unchanged (`Send_Timer_Message = 0`).  \n   - If `Main_Burner_Flag == 0`:  \n       - Cycling remains unchanged (`Send_Timer_Message = 0`).  \n\n   Stability Considerations:  \n   - Ensures the system does not enter standby unnecessarily when the burner is off.  \n   - Prevents cycling changes unless explicitly required by temperature conditions.  \n\n   -----------------------------------------------------------------\n*/"
      # "/*  \n   ------------------------- SOFTWARE NOTE -------------------------  \n   This routine checks whether a message needs to be sent to reset  \n   the water heater temperature to its factory default settings.  \n\n   `Send_Vesta_Message` States:  \n   - `0`: No action required (settings are already at factory default).  \n   - `1`: Setpoint or differential has changed from factory defaults, triggering a reset.  \n\n   Behavior:  \n   - If `Main_Burner_Flag == 1`:  \n       - Ensures `Temperature_Water_Compensated` has reached or exceeded `Setpoint_Location`.  \n       - Checks if either `Setpoint_Actual` or `Differential_Actual` deviates from factory default.  \n       - Confirms `Temperature_Water_Compensated` is valid (not zero, preventing communication errors).  \n       - If all conditions are met, `Send_Vesta_Message = 1` is triggered to restore default settings.  \n\n   Stability Considerations:  \n   - Ensures communication is stable before sending a reset command.  \n   - Prevents unnecessary messages if settings are already correct.  \n   - Avoids triggering factory reset due to minor fluctuations or transient conditions.  \n\n   -----------------------------------------------------------------\n*/"
      # "/*  \n   ------------------------- SOFTWARE NOTE -------------------------  \n   This routine controls the `Send_Vesta_Message` variable based on burner status  \n   and power mode. It determines whether to restore factory settings or  \n   adjust the burner's operation.\n\n   `Send_Vesta_Message` States:  \n   - `0`: No action required (Main Burner is OFF).  \n   - `1`: Restore factory default settings (Setpoint or Differential modified).  \n   - `2`: Command to turn the burner ON.  \n   - `3`: Command to turn the burner OFF.  \n\n   Behavior:  \n   - If `Main_Burner_Flag == 0`, no action is taken (`Send_Vesta_Message = 0`).  \n   - If `BurnerPowerMode == 0`, a check ensures that the setpoint and differential  \n     match factory defaults. If altered, `Send_Vesta_Message = 1` is triggered.  \n   - If `BurnerPowerMode == 1`:  \n       - If the burner should be ON but is currently OFF (`Burner_Status == 1 && Burner == 0`),  \n         a command (`Send_Vesta_Message = 2`) is sent to turn it ON.  \n       - If the burner should be OFF but is currently ON (`Burner_Status == 0 && Burner == 1`),  \n         a command (`Send_Vesta_Message = 3`) is sent to turn it OFF.  \n\n   Stability Considerations:  \n   - Ensures that unnecessary messages are not sent when the burner remains  \n     in its intended state.  \n   - Prevents unintended modifications when `Main_Burner_Flag == 0`.  \n   - Keeps power mode adjustments independent of factory reset checks.  \n\n   -----------------------------------------------------------------\n*/"
      # "Cycle the burner ON\nand OFF based on the\ntimer routine"
      # "If cycling is not enabled,\nverify and set the control\nto factory settings,\ntemperature and differential."
      n3 = call "Return to Normal.vi"() -> ()  [unwired: 9 in, 3 out]
      n4 = call "T2 Logic.vi"() -> ()  [unwired: 8 in, 4 out]
      n5 = call "Check Disable Mode.vi"() -> ()  [unwired: 10 in, 2 out]
      n6 = call "Function 0.vi"() -> ("error out"=w55:errorcluster, "Data Cluster Out"=w56:T3, "Send_Vesta_Message"=w57:u8, "Send_Timer_Message"=w58:u8)  [unwired: 8 in]
      n7 = call "Toggle Burner.vi"() -> ()  [unwired: 10 in, 2 out]
      n8 = call "Set to Factory Default.vi"("error in (no error)"=w55, "Send_Vesta_Message"=w57, "Data Cluster In"=w56) -> ("error out"=w53:errorcluster, "Data Cluster Out"=w54:T3)  [unwired: 7 in]
      n9 = call "Reset Timer Cycling.vi"("error in (no error)"=w53, "Send_Timer_Message"=w58, "Data Cluster In"=w54) -> ()  [unwired: 7 in, 2 out]
      n10 = case shown="False" {
        selector: _ -> [_ _]
        tunnel: [w79 w94] -> _
        tunnel: [w80 w95] -> _
        tunnel: _ -> [w78 w95]
        tunnel: _ -> [w77 w94]
        tunnel: _ -> [w81 _]
        tunnel: _ -> [w76 _]
        tunnel: _ -> [w75 _]
        frame False {
          n11 = disable-structure shown="Disabled" {
            disable-tunnel: [w90 w92] -> w84
            disable-tunnel: [w89 w93] -> w83
            disable-tunnel: [w88 u8 0 ("Send_Vesta_Message")] -> w82
            disable-tunnel: w78 -> [w87 w93]
            disable-tunnel: w77 -> [w86 w92]
            disable-tunnel: w76 -> [w85 _]
            frame Disabled {
              # "POWER MODE\n& BURNER CONTROL"
              n12 = call "Function 1.vi"("error in (no error)"=w86, "Differential_Top"=w85, "Data Cluster"=w87) -> ("error out"=w90:errorcluster, "Data Cluster Out"=w89:T3, "Send_Vesta_Message"=w88:u8)  [unwired: 6 in]
            }
            frame Enabled {
            }
          }
          n13 = call "Set to Factory Default.vi"("VestaTemperature Fixed"=w75, "error in (no error)"=w84, "Send_Vesta_Message"=w82, "Vesta in"=w81, "Data Cluster In"=w83) -> ("error out"=w79:errorcluster, "Data Cluster Out"=w80:T3)  [unwired: 5 in]
        }
        frame True {
        }
      }
      n14 = call "Enable Burner Cycle.vi"() -> ()  [unwired: 9 in, 3 out]
      n15 = call "Function 2.vi"() -> ("error out"=w47:errorcluster, "Data Cluster Out"=w46:T3, "Send_Vesta_Message"=w44:u8, "Send_Timer_Message"=w45:u8)  [unwired: 8 in]
      n16 = call "Check_Enable_Cycling_Flag.vi"() -> ("error out"=w71:errorcluster, "Data Cluster out"=w72:T3)  [unwired: 8 in, 2 out]
      n17 = call "Set to Factory Default.vi"("error in (no error)"=w71, "Data Cluster In"=w72) -> ("error out"=w73:errorcluster, "Data Cluster Out"=w74:T3)  [unwired: 8 in]
      n18 = call "Reset Timer Cycling.vi"("error in (no error)"=w73, "Data Cluster In"=w74) -> ()  [unwired: 8 in, 2 out]
      n19 = call "Enable Cycling.vi"() -> ("error out"=w68:errorcluster, "Data Cluster out"=w67:T3, "Send_Vesta_Message"=w69:u8, "Send_Timer_Message"=w70:u8)  [unwired: 8 in]
      n20 = call "PowerModeSwitch.vi"() -> ("error out"=w60:errorcluster, "Data Cluster out"=w61:T3, "Send_Vesta_Message"=w64:u8, "Send_Timer_Message"=w59:u8)  [unwired: 8 in]
      n21 = call "Set to Factory Default.vi"("error in (no error)"=w68, "Send_Vesta_Message"=w69, "Data Cluster In"=w67) -> ("error out"=w66:errorcluster, "Data Cluster Out"=w65:T3)  [unwired: 7 in]
      n22 = call "Set to Factory Default.vi"("error in (no error)"=w60, "Send_Vesta_Message"=w64, "Data Cluster In"=w61) -> ("error out"=w63:errorcluster, "Data Cluster Out"=w62:T3)  [unwired: 7 in]
      n23 = call "Reset Timer Cycling.vi"("error in (no error)"=w66, "Send_Timer_Message"=w70, "Data Cluster In"=w65) -> ()  [unwired: 7 in, 2 out]
      n24 = call "Reset Timer Cycling.vi"("error in (no error)"=w63, "Send_Timer_Message"=w59, "Data Cluster In"=w62) -> ()  [unwired: 7 in, 2 out]
      n25 = call "Set to Factory Default.vi"("error in (no error)"=w47, "Send_Vesta_Message"=w44, "Vesta in"=w52, "Data Cluster In"=w46) -> ("error out"=w49:errorcluster, "Data Cluster Out"=w48:T3)  [unwired: 6 in]
      n26 = call "Reset Timer Cycling.vi"("error in (no error)"=w49, "Send_Timer_Message"=w45, "Data Cluster In"=w48) -> ("error out"=w50:errorcluster, "Data Cluster Output"=w51:T3)  [unwired: 7 in]
      n27 = call "Function 3.vi"("error in (no error)"=w50, "Data Cluster in"=w51) -> ("error out"=w41:errorcluster, "Data Cluster 3"=w42:T3, "Send_Vesta_Message"=w43:u8)  [unwired: 7 in]
      n28 = call "Set to Factory Default.vi"("error in (no error)"=w41, "Send_Vesta_Message"=w43, "Data Cluster In"=w42) -> ("Vesta in"=w52:refnum<queue>)  [unwired: 6 in, 2 out]
    }
    frame Enabled {
    }
  }
  n29 = case shown="0, Default" w3 {
    tunnel: [TRUE FALSE] -> w4
    frame 0, Default {
    }
    frame 1 {
    }
  }
  n30 = call <vilib>:"Trim Whitespace.vi"("string"=w26, "location (both)"=w27) -> ("trimmed string"=w22:string)
  n31 = case shown="\"1F00\", \"1F1F\"" w22 {
    tunnel: [1 0] -> w21
    frame "1F00", "1F1F" {
    }
    frame "0000", "001F", Default {
    }
  }
  n32 = case shown="\"TC1\", Default" "Upper Temperature Sensor" {
    tunnel: "Data Cluster" -> [w101 w103 w105 w107 w109 w111]
    tunnel: [w100 w102 w104 w106 w108 w110] -> w20
    frame "TC1", Default {
      n33 = Unbundle By Name(w101) -> ("MW Output.TC1-Channel 021"=w100:dbl)
    }
    frame "TC2" {
      n34 = Unbundle By Name(w103) -> ("MW Output.TC2-Channel 022"=w102:dbl)
    }
    frame "TC3" {
      n35 = Unbundle By Name(w105) -> ("MW Output.TC3-Channel 023"=w104:dbl)
    }
    frame "TC4" {
      n36 = Unbundle By Name(w107) -> ("MW Output.TC4-Channel 024"=w106:dbl)
    }
    frame "TC5" {
      n37 = Unbundle By Name(w109) -> ("MW Output.TC5-Channel 025"=w108:dbl)
    }
    frame "TC6" {
      n38 = Unbundle By Name(w111) -> ("MW Output.TC6-Channel 026"=w110:dbl)
    }
  }
  n39 = call "Elapsed Time"("Time Target (s)"=10.0, "Reset"=w4, "Auto Reset"=FALSE) -> ("Elapsed Time (s)"=w2:dbl)  [unwired: 9 in, 7 out]
  n40 = case shown="\"1F00\"" w22 {
    tunnel: [0 1 2] -> w25
    frame Default {
    }
    frame "001F" {
    }
    frame "1F00" {
    }
  }
  n41 = Boolean To (0,1)(Boolean=w24) -> (0, 1=w23:i16)
  n42 = formula code="/*\n * ---------------- T2 / CYCLING / HEAT REQUEST CONTROL ----------------\n *\n * This function executes once per control-loop scan.\n *\n * OUTPUT: Send_Vesta_Message\n *\n *     0 = no Vesta command\n *     1 = restore native product control\n *     2 = force burner ON using Differential_Actual = 0.1\n *     3 = suppress burner using Setpoint_Actual = 55F\n *\n * OUTPUT: Send_Timer_Message\n *\n *     0 = no timer-state change\n *     1 = set Main_Burner_Flag TRUE\n *     5 = set Main_Burner_Flag FALSE and reset cycling state\n *\n * SAVED STATE: Off_Time_Complete_Flag\n *\n *     0 = burner has not completed the minimum OFF time\n *     1 = burner has been OFF for at least 30 seconds\n *\n * SAVED STATE: Heating_Cycle_Released_Flag\n *\n *     0 = the next heating cycle has not been released\n *     1 = native control has been released for the current cycle\n *\n * Heat_Request values:\n *\n *     0 = no recognized heat-request error\n *     1 = raw Heat Request \"001F\": burner must be turned OFF\n *     2 = raw Heat Request \"1F00\": burner must be turned ON\n *\n * Communication check:\n *\n *     Temperature_Water_Compensated == 0\n *\n *         Communication with the embedded controller has not been\n *         established. Do not send commands or change saved state.\n *\n * Normal TC2 control:\n *\n *     Stop heating when:\n *\n *         TC2 > Setpoint_Location\n *\n *     Release a new heating cycle when:\n *\n *         TC2 <= (Setpoint_Location - Differential_Top)\n *\n *     AND:\n *\n *         Off_Time_Complete_Flag == 1\n *\n * The Heating_Cycle_Released_Flag remembers that native control was\n * deliberately released. This prevents a small TC2 rebound above the\n * restart threshold from immediately returning the controller to\n * standby before the burner starts.\n *\n * Minimum OFF-time control:\n *\n *     The embedded LDO_Timer resets when the burner changes state.\n *\n *     Burner ON:\n *         Clear Off_Time_Complete_Flag.\n *\n *     Burner OFF for at least 30 seconds:\n *         Set Off_Time_Complete_Flag.\n *\n *     Once set, the flag stays set throughout the same OFF period.\n *     This prevents LDO_Timer rollover from restarting the lockout.\n *\n * Forced-ON error recovery:\n *\n *     Heat_Request == 2 applies Differential_Actual = 0.1.\n *\n *     After Heat_Request returns to zero, remove the 0.1 differential\n *     immediately. Do not wait for the TC2 restart threshold or the\n *     30-second OFF-time requirement.\n *\n * <<NEW>> Damper burner-start interlock:\n *\n *     Any command/state that can permit burner start is gated so the\n *     damper must first be commanded OPEN continuously for at least\n *     10 seconds.\n *\n *     After an actual burner cycle ends, the damper remains OPEN until\n *     LDO_Timer reaches 60 seconds.\n *\n * Control priority:\n *\n *     0. Embedded communication check\n *     1. Active Heat Request error handling\n *     2. Residual forced-ON error recovery\n *     3. Pilot position\n *     4. Normal TC2 cycle-release control\n */\n\n\n/* ---------------- Output defaults ---------------- */\n\nint32 Send_Vesta_Message = 0;\nint32 Send_Timer_Message = 0;\nint32 Open_Damper = 0;\n\n\n/* ---------------- Controller-state variables ---------------- */\n\nint32 native_controls_active = 0;\nint32 standby_is_active = 0;\nint32 forced_on_is_active = 0;\n\n\n/* ---------------- Communication and TC2 variables ---------------- */\n\nint32 lower_temperature_valid = 0;\nint32 upper_is_high = 0;\nint32 upper_restart_allowed = 0;\n\n\n/* ---------------- Previous saved-state values ---------------- */\n\nint32 Off_Time_Complete_Flag_Previous = 0;\nint32 Heating_Cycle_Released_Flag_Previous = 0;\n\n/* <<NEW>> Damper saved-state working value */\n\nint32 Damper_Burner_Seen_Flag_Previous = 0;\n\n\n/* ---------------- Constants ---------------- */\n\nfloat Pilot_Position = 0.1;\nfloat Forced_On_Differential = 0.1;\n\nint32 LDO_Timeout_OFF = 30;\n\n/* <<NEW>> Damper timing constants */\n\nint32 Damper_Preopen_Delay = 10;\nint32 Damper_Close_Delay = 60;\n\n\n/* ---------------- Decoded Heat Request values ---------------- */\n\nint32 Heat_Request_None = 0;\nint32 Heat_Request_Turn_Off = 1;  /* Raw value \"001F\" */\nint32 Heat_Request_Turn_On = 2;   /* Raw value \"1F00\" */\n\n\n/* <<NEW>> ---------------- Damper interlock working variables ---------------- */\n\nint32 Damper_Preopen_Ready = 0;\nint32 Damper_Vesta_Request = 0;\n\n\n/* ================================================================\n * SAVE INCOMING STATE VALUES\n * ================================================================ */\n\n/*\n * Both saved-state variables are Formula Node inputs and outputs.\n *\n * Preserve the incoming values by default. The control logic below\n * changes them only when a defined state transition occurs.\n */\n\nOff_Time_Complete_Flag_Previous =\n    Off_Time_Complete_Flag;\n\nHeating_Cycle_Released_Flag_Previous =\n    Heating_Cycle_Released_Flag;\n\nOff_Time_Complete_Flag =\n    Off_Time_Complete_Flag_Previous;\n\nHeating_Cycle_Released_Flag =\n    Heating_Cycle_Released_Flag_Previous;\n\n\n/* <<NEW>> ==========================================================\n * SAVE INCOMING DAMPER STATE\n * ================================================================ */\n\n/*\n * Damper_Burner_Seen_Flag is an input/output saved-state value.\n * Preserve it unless the final damper interlock changes it.\n */\n\nDamper_Burner_Seen_Flag_Previous =\n    Damper_Burner_Seen_Flag;\n\nDamper_Burner_Seen_Flag =\n    Damper_Burner_Seen_Flag_Previous;\n\n/*\n * Preserve the previous commanded damper state by default.\n */\n\nOpen_Damper = Damper_Status;\n\n\n/* ================================================================\n * DETERMINE CURRENT EMBEDDED CONTROLLER STATE\n * ================================================================ */\n\n/*\n * Native control:\n *\n *     Setpoint_Actual = physical knob setting\n *     Differential_Actual = normal embedded differential\n */\n\nnative_controls_active =\n    ((Setpoint_Actual == Setpoint_Location) &&\n     (Differential_Actual == Differential_Target)) ? 1 : 0;\n\n\n/*\n * Standby:\n *\n *     Setpoint_Actual = 55F\n *     Differential_Actual = normal embedded differential\n */\n\nstandby_is_active =\n    ((Setpoint_Actual == 55.0) &&\n     (Differential_Actual == Differential_Target)) ? 1 : 0;\n\n\n/*\n * Forced ON:\n *\n *     Setpoint_Actual = physical knob setting\n *     Differential_Actual = 0.1\n */\n\nforced_on_is_active =\n    ((Setpoint_Actual == Setpoint_Location) &&\n     (Differential_Actual == Forced_On_Differential)) ? 1 : 0;\n\n\n/* ================================================================\n * DETERMINE COMMUNICATION STATUS\n * ================================================================ */\n\n/*\n * Temperature_Water_Compensated is used only as the communication\n * check in this function.\n *\n * A value of zero indicates that a valid reading has not been\n * received from the embedded controller.\n */\n\nlower_temperature_valid =\n    (Temperature_Water_Compensated == 0) ? 0 : 1;\n\n\n/* ================================================================\n * DETERMINE TC2 CONDITIONS\n * ================================================================ */\n\n/*\n * Stop heating when TC2 rises above the physical knob setpoint.\n *\n * At exact equality, upper_is_high remains zero.\n */\n\nupper_is_high =\n    (TC2 > Setpoint_Location) ? 1 : 0;\n\n\n/*\n * Permit release of a new heating cycle after TC2 cools to or below:\n *\n *     Setpoint_Location - Differential_Top\n *\n * Example:\n *\n *     Setpoint_Location = 125F\n *     Differential_Top = 5F\n *\n *     Stop threshold:    TC2 > 125F\n *     Restart threshold: TC2 <= 120F\n */\n\nupper_restart_allowed =\n    (TC2 <=\n        (Setpoint_Location - Differential_Top)) ? 1 : 0;\n\n\n/* ================================================================\n * PRIORITY 0: EMBEDDED COMMUNICATION CHECK\n * ================================================================ */\n\nif (lower_temperature_valid == 0)\n{\n    /*\n     * Communication has not been established.\n     *\n     * Do not send Vesta commands.\n     * Do not send timer commands.\n     * Do not change either saved-state flag.\n     */\n\n    Send_Vesta_Message = 0;\n    Send_Timer_Message = 0;\n\n    Off_Time_Complete_Flag =\n        Off_Time_Complete_Flag_Previous;\n\n    Heating_Cycle_Released_Flag =\n        Heating_Cycle_Released_Flag_Previous;\n}\n\n\n/* ================================================================\n * COMMUNICATION IS VALID\n * ================================================================ */\n\nelse\n{\n    /* ------------------------------------------------------------\n     * UPDATE MINIMUM OFF-TIME STATE\n     * ------------------------------------------------------------ */\n\n    /*\n     * Burner ON:\n     *\n     * The burner is no longer in an OFF period. Clear the completed\n     * OFF-time flag.\n     */\n\n    if (Burner == 1)\n    {\n        Off_Time_Complete_Flag = 0;\n    }\n\n\n    /*\n     * Burner OFF:\n     *\n     * Set the completed flag after LDO_Timer reaches 30 seconds.\n     *\n     * Once set, preserve the flag throughout the same OFF period.\n     * LDO_Timer may later roll over, but the saved flag stays set.\n     */\n\n    else if (Burner == 0)\n    {\n        if (Off_Time_Complete_Flag_Previous == 0)\n        {\n            if (LDO_Timer >= LDO_Timeout_OFF)\n            {\n                Off_Time_Complete_Flag = 1;\n            }\n        }\n    }\n\n\n    /*\n     * Unexpected burner value:\n     *\n     * Preserve the previous OFF-time state.\n     */\n\n    else\n    {\n        Off_Time_Complete_Flag =\n            Off_Time_Complete_Flag_Previous;\n    }\n\n\n    /* ============================================================\n     * PRIORITY 1A: ACTIVE TURN-OFF ERROR\n     * ============================================================ */\n\n    /*\n     * Heat_Request == 1 corresponds to raw value \"001F\".\n     *\n     * The error condition requires the burner to be turned OFF.\n     */\n\n    if (Heat_Request == Heat_Request_Turn_Off)\n    {\n        /*\n         * Immediately command 55F standby.\n         *\n         * Vesta message 3 also restores:\n         *\n         *     Differential_Actual = Differential_Target\n         */\n\n        if (standby_is_active == 0)\n        {\n            Send_Vesta_Message = 3;\n        }\n\n        /*\n         * Withdraw normal-cycle permission.\n         *\n         * After the error clears, the next normal cycle must satisfy\n         * the TC2 restart and minimum OFF-time requirements.\n         */\n\n        Heating_Cycle_Released_Flag = 0;\n\n        /*\n         * Do not clear Main_Burner_Flag until Burner == 0 confirms\n         * that the burner has physically shut down.\n         */\n    }\n\n\n    /* ============================================================\n     * PRIORITY 1B: ACTIVE FORCED-ON ERROR\n     * ============================================================ */\n\n    /*\n     * Heat_Request == 2 corresponds to raw value \"1F00\".\n     *\n     * The error condition requires the burner to be turned ON.\n     */\n\n    else if (Heat_Request == Heat_Request_Turn_On)\n    {\n        /*\n         * Immediately apply the 0.1 embedded lower differential.\n         *\n         * Active error handling is not delayed by TC2 restart\n         * permission or the 30-second minimum OFF time.\n         */\n\n        if (forced_on_is_active == 0)\n        {\n            Send_Vesta_Message = 2;\n        }\n\n        /*\n         * Preserve Heating_Cycle_Released_Flag while the active error\n         * is present.\n         *\n         * The residual forced-ON recovery below determines the proper\n         * normal state after Heat_Request returns to zero.\n         */\n    }\n\n\n    /* ============================================================\n     * PRIORITY 2: NO ACTIVE HEAT REQUEST ERROR\n     * ============================================================ */\n\n    else if (Heat_Request == Heat_Request_None)\n    {\n        /* --------------------------------------------------------\n         * RESIDUAL FORCED-ON ERROR RECOVERY\n         * -------------------------------------------------------- */\n\n        /*\n         * Heat_Request has cleared, but the controller still reports:\n         *\n         *     Setpoint_Actual = Setpoint_Location\n         *     Differential_Actual = 0.1\n         *\n         * Remove the 0.1 differential immediately.\n         *\n         * Do not wait for:\n         *\n         *     upper_restart_allowed\n         *     Off_Time_Complete_Flag\n         */\n\n        if (forced_on_is_active == 1)\n        {\n            /*\n             * TC2 is above the customer setpoint.\n             *\n             * Enter standby immediately and withdraw heating-cycle\n             * permission.\n             */\n\n            if (upper_is_high == 1)\n            {\n                Send_Vesta_Message = 3;\n                Heating_Cycle_Released_Flag = 0;\n            }\n\n\n            /*\n             * TC2 is not above the customer setpoint.\n             *\n             * Immediately restore:\n             *\n             *     Setpoint_Actual = Setpoint_Location\n             *     Differential_Actual = Differential_Target\n             *\n             * Consider the current cycle released. The embedded lower\n             * thermistor then decides whether the burner continues,\n             * shuts off, or starts later.\n             */\n\n            else\n            {\n                Send_Vesta_Message = 1;\n                Heating_Cycle_Released_Flag = 1;\n            }\n\n\n            /*\n             * Synchronize Main_Burner_Flag with the physical burner.\n             */\n\n            if (Burner == 1)\n            {\n                if (Main_Burner_Flag == 0)\n                {\n                    Send_Timer_Message = 1;\n                }\n            }\n\n            else if (Burner == 0)\n            {\n                if (Main_Burner_Flag == 1)\n                {\n                    Send_Timer_Message = 5;\n                }\n            }\n        }\n\n\n        /* --------------------------------------------------------\n         * USER-SELECTED PILOT POSITION\n         * -------------------------------------------------------- */\n\n        else if (Setpoint_Location == Pilot_Position)\n        {\n            /*\n             * Pilot was selected using the physical product control.\n             *\n             * Do not send Vesta or timer commands.\n             * Withdraw normal heating-cycle permission so that the\n             * control initializes again after leaving Pilot.\n             */\n\n            Send_Vesta_Message = 0;\n            Send_Timer_Message = 0;\n\n            Heating_Cycle_Released_Flag = 0;\n        }\n\n\n        /* --------------------------------------------------------\n         * BURNER ON\n         * -------------------------------------------------------- */\n\n        else if (Burner == 1)\n        {\n            /*\n             * TC2 is above the physical knob setpoint.\n             *\n             * Stop heating immediately regardless of release state.\n             */\n\n            if (upper_is_high == 1)\n            {\n                if (standby_is_active == 0)\n                {\n                    Send_Vesta_Message = 3;\n                }\n\n                /*\n                 * Withdraw permission for the next heating cycle.\n                 */\n\n                Heating_Cycle_Released_Flag = 0;\n\n                /*\n                 * Do not clear Main_Burner_Flag yet.\n                 *\n                 * Wait for Burner == 0 to confirm physical shutdown.\n                 */\n            }\n\n\n            /*\n             * A normal cycle was previously released.\n             *\n             * Continue heating while TC2 remains at or below the\n             * upper stopping threshold.\n             */\n\n            else if (Heating_Cycle_Released_Flag_Previous == 1)\n            {\n                Heating_Cycle_Released_Flag = 1;\n\n                if (Main_Burner_Flag == 0)\n                {\n                    Send_Timer_Message = 1;\n                }\n            }\n\n\n            /*\n             * Burner is already ON, but no released cycle has yet\n             * been recorded.\n             *\n             * This can happen during:\n             *\n             *     Cold-tank startup\n             *     Software restart\n             *     State recovery\n             *\n             * Adopt the active cycle only when TC2 is already at or\n             * below the normal restart threshold.\n             */\n\n            else\n            {\n                if (upper_restart_allowed == 1)\n                {\n                    /*\n                     * Adopt the valid cold-start heating cycle.\n                     */\n\n                    Heating_Cycle_Released_Flag = 1;\n\n                    /*\n                     * If the controller is not already in native mode,\n                     * restore native settings.\n                     */\n\n                    if (native_controls_active == 0)\n                    {\n                        Send_Vesta_Message = 1;\n                    }\n\n                    if (Main_Burner_Flag == 0)\n                    {\n                        Send_Timer_Message = 1;\n                    }\n                }\n\n\n                /*\n                 * The burner is ON, but TC2 is still above the restart\n                 * threshold.\n                 *\n                 * Do not adopt this cycle. Command standby and keep the\n                 * cycle locked out.\n                 */\n\n                else\n                {\n                    if (standby_is_active == 0)\n                    {\n                        Send_Vesta_Message = 3;\n                    }\n\n                    Heating_Cycle_Released_Flag = 0;\n                }\n            }\n        }\n\n\n        /* --------------------------------------------------------\n         * BURNER OFF\n         * -------------------------------------------------------- */\n\n        else if (Burner == 0)\n        {\n            /*\n             * Clear Main_Burner_Flag only after physical burner\n             * shutdown is confirmed.\n             */\n\n            if (Main_Burner_Flag == 1)\n            {\n                Send_Timer_Message = 5;\n            }\n\n\n            /*\n             * A cycle was previously released.\n             */\n\n            if (Heating_Cycle_Released_Flag_Previous == 1)\n            {\n                /*\n                 * TC2 has exceeded the customer setpoint while the\n                 * burner is OFF.\n                 *\n                 * Enter standby and close the released cycle.\n                 */\n\n                if (upper_is_high == 1)\n                {\n                    if (standby_is_active == 0)\n                    {\n                        Send_Vesta_Message = 3;\n                    }\n\n                    Heating_Cycle_Released_Flag = 0;\n                }\n\n\n                /*\n                 * Main_Burner_Flag is still one while Burner is zero.\n                 *\n                 * The embedded controller has just ended an active\n                 * burner cycle. Enter standby and require the next\n                 * cycle to satisfy TC2 and minimum OFF-time criteria.\n                 */\n\n                else if (Main_Burner_Flag == 1)\n                {\n                    if (standby_is_active == 0)\n                    {\n                        Send_Vesta_Message = 3;\n                    }\n\n                    Heating_Cycle_Released_Flag = 0;\n                }\n\n\n                /*\n                 * The cycle has been released, but the burner has not\n                 * started yet.\n                 *\n                 * Keep native control released while waiting for the\n                 * embedded lower thermistor to call for heat.\n                 *\n                 * Do not cancel the release merely because TC2 rises\n                 * slightly above the restart threshold.\n                 */\n\n                else\n                {\n                    Heating_Cycle_Released_Flag = 1;\n\n                    /*\n                     * If message 1 has not yet been acknowledged and\n                     * standby still reports active, repeat the same\n                     * release command. Do not issue an opposing\n                     * standby command.\n                     */\n\n                    if (standby_is_active == 1)\n                    {\n                        Send_Vesta_Message = 1;\n                    }\n\n                    else\n                    {\n                        Send_Vesta_Message = 0;\n                    }\n                }\n            }\n\n\n            /*\n             * No heating cycle is currently released.\n             */\n\n            else\n            {\n                /*\n                 * TC2 is above the physical knob setpoint.\n                 *\n                 * Ensure the controller is in standby.\n                 */\n\n                if (upper_is_high == 1)\n                {\n                    if (standby_is_active == 0)\n                    {\n                        Send_Vesta_Message = 3;\n                    }\n\n                    Heating_Cycle_Released_Flag = 0;\n                }\n\n\n                /*\n                 * The controller already reports standby.\n                 *\n                 * Release native control only after:\n                 *\n                 *     1. TC2 reaches the restart threshold.\n                 *     2. Burner has been OFF for at least 30 seconds.\n                 */\n\n                else if (standby_is_active == 1)\n                {\n                    if ((upper_restart_allowed == 1) &&\n                        (Off_Time_Complete_Flag == 1))\n                    {\n                        Send_Vesta_Message = 1;\n                        Heating_Cycle_Released_Flag = 1;\n                    }\n\n                    else\n                    {\n                        Send_Vesta_Message = 0;\n                        Heating_Cycle_Released_Flag = 0;\n                    }\n                }\n\n\n                /*\n                 * The controller reports native mode, but the cycle\n                 * has not yet been released.\n                 *\n                 * This is the startup and state-initialization case.\n                 */\n\n                else if (native_controls_active == 1)\n                {\n                    /*\n                     * Cold start or sufficiently cooled tank:\n                     *\n                     * Native control may remain active only after the\n                     * TC2 and minimum OFF-time criteria are satisfied.\n                     */\n\n                    if ((upper_restart_allowed == 1) &&\n                        (Off_Time_Complete_Flag == 1))\n                    {\n                        Send_Vesta_Message = 0;\n                        Heating_Cycle_Released_Flag = 1;\n                    }\n\n\n                    /*\n                     * Hot startup or minimum OFF time not complete:\n                     *\n                     * Place the controller into standby and lock out\n                     * the next heating cycle.\n                     */\n\n                    else\n                    {\n                        Send_Vesta_Message = 3;\n                        Heating_Cycle_Released_Flag = 0;\n                    }\n                }\n\n\n                /*\n                 * The applied state does not match native or standby.\n                 *\n                 * This may occur while a previous Vesta command is\n                 * still being processed. Do not issue an opposing\n                 * command.\n                 */\n\n                else\n                {\n                    Send_Vesta_Message = 0;\n                    Heating_Cycle_Released_Flag = 0;\n                }\n            }\n        }\n\n\n        /* --------------------------------------------------------\n         * UNEXPECTED BURNER VALUE\n         * -------------------------------------------------------- */\n\n        else\n        {\n            Send_Vesta_Message = 0;\n            Send_Timer_Message = 0;\n\n            Heating_Cycle_Released_Flag =\n                Heating_Cycle_Released_Flag_Previous;\n        }\n    }\n\n\n    /* ============================================================\n     * UNEXPECTED HEAT REQUEST VALUE\n     * ============================================================ */\n\n    else\n    {\n        Send_Vesta_Message = 0;\n        Send_Timer_Message = 0;\n\n        Heating_Cycle_Released_Flag =\n            Heating_Cycle_Released_Flag_Previous;\n    }\n}\n\n\n/* <<NEW>> ==========================================================\n * FINAL DAMPER / BURNER-START INTERLOCK\n * ================================================================ */\n\n/*\n * IMPORTANT:\n *\n * The existing heater-control logic above is intentionally left\n * unchanged. It calculates Send_Vesta_Message and the heater saved\n * states exactly as before.\n *\n * This final block gates any condition that can permit burner start.\n *\n * Requirement:\n *\n *     The damper must be commanded OPEN continuously for at least\n *     Damper_Preopen_Delay seconds before burner start is permitted.\n *\n * Damper_Open_Timer is an INPUT to this Formula Node.\n * It must measure continuous commanded-open time:\n *\n *     Open_Damper = 0  -> timer reset to 0\n *     Open_Damper = 1  -> timer counts upward in seconds\n *\n * A new heating request while the damper is already OPEN for at least\n * 10 seconds does not require the damper to close and reopen.\n *\n * After an actual burner cycle, Damper_Burner_Seen_Flag remains set\n * until the 60-second post-purge is complete.\n */\n\n\n/* ------------------------------------------------------------\n * CAPTURE THE VESTA COMMAND REQUESTED BY THE EXISTING LOGIC\n * ------------------------------------------------------------ */\n\nDamper_Vesta_Request = Send_Vesta_Message;\n\n\n/* ------------------------------------------------------------\n * DETERMINE WHETHER 10-SECOND PRE-OPEN IS COMPLETE\n * ------------------------------------------------------------ */\n\n/*\n * Damper_Status is the saved commanded state from the previous scan.\n * Requiring Damper_Status == 1 prevents the same scan that first\n * commands OPEN from also satisfying the pre-open requirement.\n */\n\nDamper_Preopen_Ready =\n    ((Damper_Status == 1) &&\n     (Damper_Open_Timer >= Damper_Preopen_Delay)) ? 1 : 0;\n\n\n/* ------------------------------------------------------------\n * COMMUNICATION NOT ESTABLISHED\n * ------------------------------------------------------------ */\n\nif (lower_temperature_valid == 0)\n{\n    /*\n     * Existing heater logic already sets:\n     *\n     *     Send_Vesta_Message = 0\n     *     Send_Timer_Message = 0\n     *\n     * while preserving heater saved state.\n     *\n     * Do the same for the damper: make no new decision and preserve\n     * both saved damper states.\n     */\n\n    Open_Damper = Damper_Status;\n\n    Damper_Burner_Seen_Flag =\n        Damper_Burner_Seen_Flag_Previous;\n}\n\n\n/* ------------------------------------------------------------\n * COMMUNICATION IS VALID\n * ------------------------------------------------------------ */\n\nelse\n{\n    /* --------------------------------------------------------\n     * BURNER IS PHYSICALLY ON\n     * -------------------------------------------------------- */\n\n    if (Burner == 1)\n    {\n        /*\n         * Burner is physically operating.\n         * Keep the damper OPEN and remember that the burner ran.\n         *\n         * NOTE:\n         * This cannot retroactively satisfy the 10-second pre-open\n         * requirement if software is started with Burner already ON.\n         */\n\n        Open_Damper = 1;\n        Damper_Burner_Seen_Flag = 1;\n    }\n\n\n    /* --------------------------------------------------------\n     * BURNER IS PHYSICALLY OFF\n     * -------------------------------------------------------- */\n\n    else if (Burner == 0)\n    {\n        /* <<NEW - PILOT FIX>> ---------------------------------\n         * PILOT POSITION\n         * ---------------------------------------------------- */\n\n        /*\n         * The existing heater logic treats Pilot as a special\n         * non-heating state.\n         *\n         * While in Pilot:\n         *\n         *     Setpoint_Actual may equal Setpoint_Location\n         *\n         * which can cause:\n         *\n         *     native_controls_active == 1\n         *\n         * The damper interlock must NOT interpret that Pilot\n         * condition as a burner-start-capable native state.\n         *\n         * Active Heat Request errors retain higher priority.\n         * Therefore this Pilot branch applies only when:\n         *\n         *     Heat_Request == Heat_Request_None\n         */\n\n        if ((Heat_Request == Heat_Request_None) &&\n            (Setpoint_Location == Pilot_Position))\n        {\n            /*\n             * Preserve the existing heater Pilot behavior.\n             */\n\n            Send_Vesta_Message = 0;\n            Heating_Cycle_Released_Flag = 0;\n\n\n            /* <<NEW - PILOT TIMER FIX>>\n             *\n             * This branch is already inside Burner == 0.\n             *\n             * If an actual burner cycle occurred and\n             * Main_Burner_Flag is still set, send Timer 5\n             * so the burner-cycle timing state can clear\n             * and the normal 60-second post-purge can complete.\n             */\n\n            if ((Damper_Burner_Seen_Flag_Previous == 1) &&\n                (Main_Burner_Flag == 1))\n            {\n                Send_Timer_Message = 5;\n            }\n\n            else\n            {\n                Send_Timer_Message = 0;\n            }\n\n\n            /*\n             * If an actual burner cycle occurred before entering\n             * Pilot, preserve the normal 60-second post-purge.\n             */\n\n            if (Damper_Burner_Seen_Flag_Previous == 1)\n            {\n                Open_Damper = 1;\n\n\n                /*\n                 * Close only after:\n                 *\n                 *     Main_Burner_Flag has been cleared\n                 *\n                 * AND\n                 *\n                 *     LDO_Timer has reached 60 seconds.\n                 */\n\n                if ((Main_Burner_Flag == 0) &&\n                    (LDO_Timer >= Damper_Close_Delay))\n                {\n                    Open_Damper = 0;\n                    Damper_Burner_Seen_Flag = 0;\n                }\n            }\n\n\n            /*\n             * No burner cycle occurred.\n             *\n             * Pilot does not require the damper to remain OPEN.\n             */\n\n            else\n            {\n                Open_Damper = 0;\n                Damper_Burner_Seen_Flag = 0;\n            }\n        }\n\n\n        /* ----------------------------------------------------\n         * VESTA 3: SUPPRESS / TURN-OFF COMMAND\n         * ---------------------------------------------------- */\n\n        else if (Damper_Vesta_Request == 3)\n        {\n            /*\n             * A suppress command never permits a burner start, so it\n             * must never be blocked by the damper pre-open interlock.\n             *\n             * If a burner actually ran, preserve the damper through\n             * the post-purge. Otherwise the damper may close.\n             */\n\n            if (Damper_Burner_Seen_Flag_Previous == 1)\n            {\n                Open_Damper = 1;\n\n                if ((Main_Burner_Flag == 0) &&\n                    (LDO_Timer >= Damper_Close_Delay))\n                {\n                    Open_Damper = 0;\n                    Damper_Burner_Seen_Flag = 0;\n                }\n            }\n\n            else\n            {\n                Open_Damper = 0;\n                Damper_Burner_Seen_Flag = 0;\n            }\n        }\n\n\n        /* ----------------------------------------------------\n         * VESTA 1 OR 2: BURNER-START-ENABLING COMMAND PENDING\n         * ---------------------------------------------------- */\n\n        else if ((Damper_Vesta_Request == 1) ||\n                 (Damper_Vesta_Request == 2))\n        {\n            /*\n             * Vesta 1 restores native product control.\n             * Vesta 2 applies the forced-ON differential.\n             *\n             * Either command can permit the burner to start.\n             * Command the damper OPEN first.\n             */\n\n            Open_Damper = 1;\n\n\n            /*\n             * Block the requested Vesta command until the damper has\n             * been continuously commanded OPEN for at least 10 seconds.\n             */\n\n            if (Damper_Preopen_Ready == 0)\n            {\n                /*\n                 * If the existing logic attempted to release a normal\n                 * cycle with Vesta 1, do not record that cycle as\n                 * released until Vesta 1 is actually allowed through.\n                 */\n\n                if (Damper_Vesta_Request == 1)\n                {\n                    Heating_Cycle_Released_Flag = 0;\n                }\n\n\n                /*\n                 * Normally, simply suppress the pending Vesta command.\n                 *\n                 * If the embedded controller already reports native or\n                 * forced-ON mode, send Vesta 3 instead so it cannot remain\n                 * in a burner-start-capable state while the 10-second\n                 * damper pre-open is still incomplete.\n                 */\n\n                if ((native_controls_active == 1) ||\n                    (forced_on_is_active == 1))\n                {\n                    Send_Vesta_Message = 3;\n                }\n\n                else\n                {\n                    Send_Vesta_Message = 0;\n                }\n            }\n\n            /*\n             * If Damper_Preopen_Ready == 1, do not modify\n             * Send_Vesta_Message. The existing Vesta 1 or 2 request is\n             * allowed through unchanged.\n             */\n        }\n\n\n        /* ----------------------------------------------------\n         * BURNER-START-CAPABLE STATE ALREADY EXISTS\n         * ---------------------------------------------------- */\n\n        else if ((Heating_Cycle_Released_Flag == 1) ||\n                 (native_controls_active == 1) ||\n                 (forced_on_is_active == 1))\n        {\n            /*\n             * Native control has already been released, or the embedded\n             * controller already reports a state that could start the\n             * burner. The damper must remain OPEN.\n             */\n\n            Open_Damper = 1;\n\n\n            /*\n             * If this state exists before the 10-second pre-open is\n             * complete, force standby and withdraw normal-cycle release.\n             *\n             * This also protects the existing native-mode startup path,\n             * which can otherwise remain native without issuing a new\n             * Vesta 1 command.\n             */\n\n            if (Damper_Preopen_Ready == 0)\n            {\n                Send_Vesta_Message = 3;\n                Heating_Cycle_Released_Flag = 0;\n            }\n        }\n\n\n        /* ----------------------------------------------------\n         * POST-PURGE AFTER AN ACTUAL BURNER CYCLE\n         * ---------------------------------------------------- */\n\n        else if (Damper_Burner_Seen_Flag_Previous == 1)\n        {\n            /*\n             * Burner has operated during this damper-open period.\n             * Keep the damper OPEN while LDO_Timer counts the physical\n             * burner-OFF period.\n             */\n\n            Open_Damper = 1;\n\n\n            /*\n             * Close after 60 seconds of burner OFF time.\n             *\n             * A new Vesta 1 or 2 request above has higher priority, so a\n             * new cycle will keep the damper OPEN rather than close it.\n             */\n\n            if ((Main_Burner_Flag == 0) &&\n                (LDO_Timer >= Damper_Close_Delay))\n            {\n                Open_Damper = 0;\n                Damper_Burner_Seen_Flag = 0;\n            }\n        }\n\n\n        /* ----------------------------------------------------\n         * NO ACTIVE OR PENDING BURNER CYCLE\n         * ---------------------------------------------------- */\n\n        else\n        {\n            Open_Damper = 0;\n            Damper_Burner_Seen_Flag = 0;\n        }\n    }\n\n\n    /* --------------------------------------------------------\n     * UNEXPECTED BURNER VALUE\n     * -------------------------------------------------------- */\n\n    else\n    {\n        Open_Damper = Damper_Status;\n\n        Damper_Burner_Seen_Flag =\n            Damper_Burner_Seen_Flag_Previous;\n    }\n}\n\n\n/* <<NEW>> ==========================================================\n * SAVE COMMANDED DAMPER STATE FOR NEXT SCAN\n * ================================================================ */\n\nDamper_Status = Open_Damper;"("Temperature_Water_Compensated"=w36, "Setpoint_Location"=w31, "Setpoint_Actual"=w30, "Differential_Actual"=w29, "Differential_Target"=w28, "TC2"=w20, "Heat_Request"=w25, "Main_Burner_Flag"=w23, "Burner"=w21, "Differential_Top"="Differential_Top", "LDO_Timer"=w19, "Off_Time_Complete_Flag"=w18, "Heating_Cycle_Released_Flag"=w14, "Damper_Status"=w3, "Damper_Burner_Seen_Flag"=w9, "Damper_Open_Timer"=w2) -> ("Send_Vesta_Message"=w33:i32, "Send_Timer_Message"=w32:i32, "Off_Time_Complete_Flag"=w15:u8, "Heating_Cycle_Released_Flag"=w13:u8, "Damper_Status"=w10:u8, "Damper_Burner_Seen_Flag"=w8:u8, "Open_Damper"=→"Open_Damper":i32)
  n43 = Bundle By Name(cluster="Data Cluster", "Timer Application Data.Duty Cycle.Damper Burner Seen Flag"=w8, "Timer Application Data.Duty Cycle.Damper Status"=w10, "Timer Application Data.Duty Cycle.Heating_Cycle_Released_Flag"=w13, "Timer Application Data.Duty Cycle.Off Time Complete Flag"=w15) -> (w16:T3)
  n44 = call "Set to Factory Default.vi"("VestaTemperature Fixed"="VestaTemperature Fixed", "error in (no error)"="error in (no error)", "Send_Vesta_Message"=w33, "Vesta in"="Vesta in", "Data Cluster In"=w16) -> ("error out"=w34:errorcluster, "Data Cluster Out"=w35:T3)  [unwired: 5 in]
  n45 = call "Reset Timer Cycling.vi"("error in (no error)"=w34, "Send_Timer_Message"=w32, "Data Cluster In"=w35) -> ("error out"=→"error out":errorcluster, "Data Cluster Output"=→"Data Cluster Output":T3)  [unwired: 7 in]
  n46 = disable-structure shown="Disabled" {
    frame Disabled {
      w124 = T9 0 items=["both", "start of string", "end of string"] ("location (both)")
      n47 = Unbundle By Name() -> ("Vesta Data Output.Temperature Water Compensated (F)"=w115:dbl, "Timer Application Data.Duty Cycle.Heating_Cycle_Released_Flag"=w116:u8, "Timer Application Data.Duty Cycle.Damper Burner Seen Flag"=w117:u8, "Timer Application Data.Duty Cycle.Damper Status"=w118:u8, "Vesta Data Output.LDO Timer (sec)"=w120:i16, "Vesta Data Output.Setpoint Location (F)"=w119:dbl, "Vesta Data Output.Heat Request"=w122:string)  [unwired: 1 in]
      n48 = call <vilib>:"Trim Whitespace.vi"("string"=w122, "location (both)"=w124) -> ("trimmed string"=w123:string)
      n49 = case shown="\"1F00\", \"1F1F\"" w123 {
        tunnel: [1 0] -> w121
        frame "1F00", "1F1F" {
        }
        frame "0000", "001F", Default {
        }
      }
      n50 = formula code="/*\n * ---------------- DAMPER CONTROL ----------------\n *\n * This control does not modify the existing TC2 / Vesta burner\n * cycling logic. It reads existing heater state as needed to\n * coordinate damper operation.\n *\n *\n * OUTPUT: Open_Damper\n *\n *     0 = command damper CLOSED\n *     1 = command damper OPEN\n *\n *\n * INPUT / OUTPUT SAVED STATE: Damper_Status\n *\n *     Previous/current commanded damper state.\n *\n *     0 = damper commanded CLOSED\n *     1 = damper commanded OPEN\n *\n *     Incoming Damper_Status contains the commanded state from\n *     the previous control-loop scan.\n *\n *     At the end of this function:\n *\n *         Damper_Status = Open_Damper;\n *\n *     saves the newly calculated state for the next scan.\n *\n *     Initialize Damper_Status to 0 when the software starts.\n *\n *\n * INPUT / OUTPUT SAVED STATE: Damper_Burner_Seen_Flag\n *\n *     0 = burner has not operated since this damper-open event\n *     1 = burner has operated since this damper-open event\n *\n *     This flag must be retained between control-loop scans.\n *     Initialize it to 0 when the software starts.\n *\n *\n * COMMUNICATION CHECK:\n *\n *     Temperature_Water_Compensated == 0\n *\n *         Communication with the embedded controller has not been\n *         established.\n *\n *         Do not make a new damper-control decision.\n *         Preserve Damper_Status.\n *         Preserve Damper_Burner_Seen_Flag.\n *\n *     Temperature_Water_Compensated != 0\n *\n *         Communication is valid and normal damper control\n *         is permitted.\n *\n *\n * NORMAL DAMPER PRE-OPEN:\n *\n *     Existing normal native-control release occurs when:\n *\n *         TC2 <= (Setpoint_Location - Differential_Top)\n *\n *     AND:\n *\n *         Off_Time_Complete_Flag == 1\n *\n *     The damper is commanded OPEN slightly BEFORE this TC2\n *     release point:\n *\n *         TC2 <= (Setpoint_Location\n *                 - Differential_Top\n *                 + Damper_Open_Lead)\n *\n *\n * Example:\n *\n *     Setpoint_Location = 125F\n *     Differential_Top = 5F\n *     Damper_Open_Lead  = 1F\n *\n *     Damper pre-open:       TC2 <= 121F\n *     Native cycle release:  TC2 <= 120F\n *\n *\n * STARTUP:\n *\n *     Damper control is disabled until embedded communication\n *     has been established.\n *\n *     If the burner is already operating when communication\n *     becomes valid:\n *\n *         Command damper OPEN immediately.\n *         Set Damper_Burner_Seen_Flag = 1.\n *\n *\n * DAMPER HOLD:\n *\n *     Once the damper opens, keep it OPEN while waiting for the\n *     burner and throughout the complete burner cycle.\n *\n *     When Burner == 1:\n *\n *         Damper_Burner_Seen_Flag = 1\n *\n *     This remembers that the burner actually operated during\n *     this damper-open period.\n *\n *\n * POST-PURGE:\n *\n *     After Burner changes to OFF, the existing LDO_Timer resets\n *     and begins counting upward.\n *\n *     Do not close the damper until:\n *\n *         Burner == 0\n *\n *     AND:\n *\n *         Damper_Burner_Seen_Flag == 1\n *\n *     AND:\n *\n *         LDO_Timer >= Damper_Close_Delay\n *\n *     AND:\n *\n *         Heating_Cycle_Released_Flag == 0\n *\n *     AND:\n *\n *         TC2 > Damper_Open_Threshold\n *\n *\n *     Heating_Cycle_Released_Flag == 0 prevents closing the damper\n *     while native control is still released and the burner could\n *     potentially start.\n *\n *     TC2 > Damper_Open_Threshold prevents closing the damper only\n *     to reopen it immediately on the next scan because TC2 is\n *     already within the damper pre-open region.\n *\n *\n *     After the post-purge is complete:\n *\n *         Open_Damper = 0\n *         Damper_Burner_Seen_Flag = 0\n *\n *     The damper is then ready for the next cycle.\n */\n\n\n/* ---------------- Constants ---------------- */\n\nfloat Damper_Open_Lead = 1.0;\n\nint32 Damper_Close_Delay = 60;\n\n\n/* ---------------- Damper working variables ---------------- */\n\nfloat Damper_Open_Threshold = 0.0;\n\nint32 Damper_Burner_Seen_Flag_Previous = 0;\n\nint32 lower_temperature_valid = 0;\n\n\n/* ---------------- Output ---------------- */\n\nint32 Open_Damper = 0;\n\n\n/* ================================================================\n * SAVE INCOMING DAMPER STATE\n * ================================================================ */\n\n/*\n * Save the incoming burner-seen state from the previous scan.\n */\n\nDamper_Burner_Seen_Flag_Previous =\n    Damper_Burner_Seen_Flag;\n\n\n/*\n * Preserve the previous value unless a defined transition below\n * changes it.\n */\n\nDamper_Burner_Seen_Flag =\n    Damper_Burner_Seen_Flag_Previous;\n\n\n/* ================================================================\n * DETERMINE COMMUNICATION STATUS\n * ================================================================ */\n\n/*\n * Temperature_Water_Compensated is used only as the communication\n * check in this damper-control function.\n *\n * A value of zero indicates that valid communication with the\n * embedded controller has not yet been established.\n */\n\nlower_temperature_valid =\n    (Temperature_Water_Compensated == 0) ? 0 : 1;\n\n\n/* ================================================================\n * CALCULATE DAMPER PRE-OPEN THRESHOLD\n * ================================================================ */\n\n/*\n * Example:\n *\n *     125F setpoint\n *     - 5F Differential_Top\n *     + 1F Damper_Open_Lead\n *\n *     = 121F damper-open threshold\n */\n\nDamper_Open_Threshold =\n    Setpoint_Location\n    - Differential_Top\n    + Damper_Open_Lead;\n\n\n/* ================================================================\n * OUTPUT DEFAULT\n * ================================================================ */\n\n/*\n * Preserve the previous commanded damper state unless a defined\n * OPEN or CLOSE transition occurs.\n */\n\nOpen_Damper = Damper_Status;\n\n\n/* ================================================================\n * PRIORITY 0: EMBEDDED COMMUNICATION CHECK\n * ================================================================ */\n\nif (lower_temperature_valid == 0)\n{\n    /*\n     * Communication has not been established.\n     *\n     * Do not make a new damper-control decision.\n     * Preserve the previous commanded damper state.\n     * Preserve the previous burner-seen state.\n     */\n\n    Open_Damper = Damper_Status;\n\n    Damper_Burner_Seen_Flag =\n        Damper_Burner_Seen_Flag_Previous;\n}\n\n\n/* ================================================================\n * COMMUNICATION IS VALID\n * ================================================================ */\n\nelse\n{\n    /* ------------------------------------------------------------\n     * PRIORITY 1: BURNER IS PHYSICALLY ON\n     * ------------------------------------------------------------ */\n\n    /*\n     * If the burner is operating, the damper must remain OPEN.\n     *\n     * This also handles the case where the burner is already ON\n     * when communication becomes valid.\n     */\n\n    if (Burner == 1)\n    {\n        Open_Damper = 1;\n\n        /*\n         * Remember that an actual burner cycle has occurred.\n         */\n\n        Damper_Burner_Seen_Flag = 1;\n    }\n\n\n    /* ------------------------------------------------------------\n     * PRIORITY 2: BURNER IS PHYSICALLY OFF\n     * ------------------------------------------------------------ */\n\n    else if (Burner == 0)\n    {\n        /* --------------------------------------------------------\n         * DAMPER CURRENTLY CLOSED\n         * -------------------------------------------------------- */\n\n        if (Damper_Status == 0)\n        {\n            /*\n             * A closed damper begins a new damper cycle.\n             *\n             * No burner operation has yet occurred for the new\n             * damper-open event.\n             */\n\n            Damper_Burner_Seen_Flag = 0;\n\n\n            /*\n             * PRE-OPEN DAMPER\n             *\n             * Open before the existing TC2 logic reaches the normal\n             * native-control release threshold.\n             */\n\n            if (TC2 <= Damper_Open_Threshold)\n            {\n                Open_Damper = 1;\n\n                /*\n                 * Burner has not started yet.\n                 *\n                 * Keep Burner_Seen zero so an old/high LDO_Timer\n                 * cannot immediately close the newly opened damper.\n                 */\n\n                Damper_Burner_Seen_Flag = 0;\n            }\n\n            else\n            {\n                Open_Damper = 0;\n            }\n        }\n\n\n        /* --------------------------------------------------------\n         * DAMPER CURRENTLY OPEN\n         * -------------------------------------------------------- */\n\n        else\n        {\n            /*\n             * Default behavior while in the OPEN state:\n             *\n             * Keep the damper OPEN.\n             */\n\n            Open_Damper = 1;\n\n\n            /*\n             * POST-PURGE CLOSE\n             *\n             * Damper may close only after:\n             *\n             *     1. Burner actually operated.\n             *     2. Burner is now OFF.\n             *     3. LDO_Timer has reached the post-purge time.\n             *     4. No heating cycle is currently released.\n             *     5. TC2 is no longer in the pre-open region.\n             */\n\n            if ((Damper_Burner_Seen_Flag_Previous == 1) &&\n                (LDO_Timer >= Damper_Close_Delay) &&\n                (Heating_Cycle_Released_Flag == 0) &&\n                (TC2 > Damper_Open_Threshold))\n            {\n                Open_Damper = 0;\n\n                /*\n                 * Post-purge is complete.\n                 *\n                 * Reset the burner-seen latch for the next\n                 * damper cycle.\n                 */\n\n                Damper_Burner_Seen_Flag = 0;\n            }\n        }\n    }\n\n\n    /* ------------------------------------------------------------\n     * UNEXPECTED BURNER VALUE\n     * ------------------------------------------------------------ */\n\n    else\n    {\n        /*\n         * Do not make a new damper decision from an invalid Burner\n         * value.\n         *\n         * Preserve both commanded state and burner-seen state.\n         */\n\n        Open_Damper = Damper_Status;\n\n        Damper_Burner_Seen_Flag =\n            Damper_Burner_Seen_Flag_Previous;\n    }\n}\n\n\n/* ================================================================\n * SAVE COMMANDED DAMPER STATE FOR NEXT SCAN\n * ================================================================ */\n\n/*\n * Store the newly calculated commanded damper state in the\n * feedback value for the next control-loop scan.\n */\n\nDamper_Status = Open_Damper;"("Burner"=w121, "LDO_Timer"=w120, "Setpoint_Location"=w119, "Damper_Status"=w118, "Damper_Burner_Seen_Flag"=w117, "Heating_Cycle_Released_Flag"=w116, "Temperature_Water_Compensated"=w115) -> ()  [unwired: 2 in, 3 out]
    }
    frame Enabled {
    }
  }
